vi "AlliGator Load IRFs & Fit Data (Map) HDF5 File v0.6.vi"(8 "Error In":errorcluster, 9 "File Type & Version only":bool, 11 "File Path":path) -> (0 "error out":errorcluster, 1 "Data Description":string, 2 "Decay Fit Options & Parameters":T1={"SYNC Period"=0.0, "Fit Options"={"Show Fit Residuals"=FALSE, "Fit Model"=enum."1-Exponential", "Residual Type"=enum."Standard", "Max Decay Percentile"=0.0, "Min Decay Percentile"=0.0, "Show Full Decay"=FALSE, "Weights"=enum."Unweighted", "Fitting Method"=enum."Least Square", "Compute Parameter Uncertainties"=FALSE, "Periodic Boundaries"=FALSE, "Model Calculation"=enum."Simulation", "Period"=0.0, "Termination Criteria"={"Max Iterations"=0, "Max Function Calls"=0, "Max Time"=0.0, "Function Tolerance"=0.0, "Parameter Tolerance"=0.0, "Gradient Tolerance"=0.0, "Min Lambda"=0.0, "Max Lambda"=0.0, "Initial Tick Count"=0}, "Offset Resolution"=0.0, "Use Local IRF"=FALSE, "Fitting Algorithm"=enum."Levenberg-Marquardt", "Show Confidence Interval "=TRUE, "Confidence Level"=95.0}, "Fit Parameter Constraints"=[], "MLE Baseline Offset"=0.0, "MLE Baseline Offset Type"=enum."Absolute"} {"Fit Options"."Confidence Level" min=0.0 max=100.0; "Fit Options"."Offset Resolution" min=0.0; "Fit Options"."Period" min=0.0; "Fit Options"."Min Decay Percentile" min=0.0 max=1.0; "Fit Options"."Max Decay Percentile" min=0.0 max=100.0; "Fit Parameter Constraints"."Max Value" format="%#.3g"; "Fit Parameter Constraints"."Min Value" format="%#.3g"}, 3 "IRFs & Fit Data Map v3":T13 {"Fit Options: Decay Preprocessing Parameters"."# Folds" min=1}, 4 "[Multiple Decays Fit Parameters SDV]":dbl[][](array[numeric]), 5 "File Version":string, 7 "File Type":string)   [LabVIEW 2021, in "AlliGator Decay Fit Parameter Map.lvlib"]
doc: "Loads Decay Fit Parameter Map and associated metadata."
uses:
  AlliGator Decay Fit Parameter Map.lvlib
  Fits/IRF(X)PSED/Decay Fit Parameters & Derived Quantities List v2.ctl
  Decay Analysis/Decay Preprocessing/AlliGator Decay Preprocessing Parameters.ctl
  Graphs/XY Graph/XY Graph Plot Shift Parameters.ctl
  Graphs/XY Graph/XY Graph Plot Shift Method.ctl
  AlliGator Decay Fit Options & Parameters v3.ctl
  Fits/IRF(X)PSED/Decay Fit Options v3.ctl
  Fits/Decay Convolution/Decay Model.ctl
  Fits/Residual Type.ctl
  Fits/IRF(X)PSED/Fit Weights Type.ctl
  Fits/Non-linear Fitting Method v2.ctl
  Fits/Fit Calculation Method.ctl
  Fits/Non-linear Fitting Algorithm.ctl
  Decay Analysis/Decay Fit/AlliGator Decay Fit Parameter Constraints 2.ctl
  Fits/IRF(X)PSED/Decay Fit Parameters In List.ctl
  Fits/IRF(X)PSED/MLE Baseline Offset Type.ctl
  Fits/IRF(X)PSED/Decay Fit Options v1.ctl
  Fits/Non-linear Fitting Method v1.ctl
  AlliGator IRFs & Fit Data v1.ctl
  Decay Analysis/Decay Fit/AlliGator Decay Fit Options & Parameters v1.ctl
  AlliGator Decay Fit Options & Parameters v2.ctl
  Fits/IRF(X)PSED/Decay Fit Options v2.ctl
  <vilib>/addons/h5labview2/base/lib_path.vi
  <vilib>/addons/h5labview2/base/H5Equery.vi
  <vilib>/addons/h5labview2/base/hid_t.ctl
  <vilib>/addons/h5labview2/dataset/H5Dread.llb/H5Dread.xnode
  <vilib>/addons/h5labview2/file/H5F.lvlib
  <vilib>/addons/h5labview2/group/H5G.lvlib
  Time/Time.lvlib
  Fits/Fits.lvlib
  Strings/Strings.lvlib
  Decay Analysis/Decay Fit/AlliGator Decay Fit.lvlib
  Graphs/XY Graph/XY Graph Add-Ons.lvlib
  Decay Analysis/Decay Preprocessing/AlliGator Decay Preprocessing.lvlib
  AlliGator IRFs & Fit Data v2.ctl
  AlliGator IRFs & Fit Data v3.ctl
panel:
  in  "Fit Parameter":T12(ring)
  out "elapsed (relative) seconds":dbl
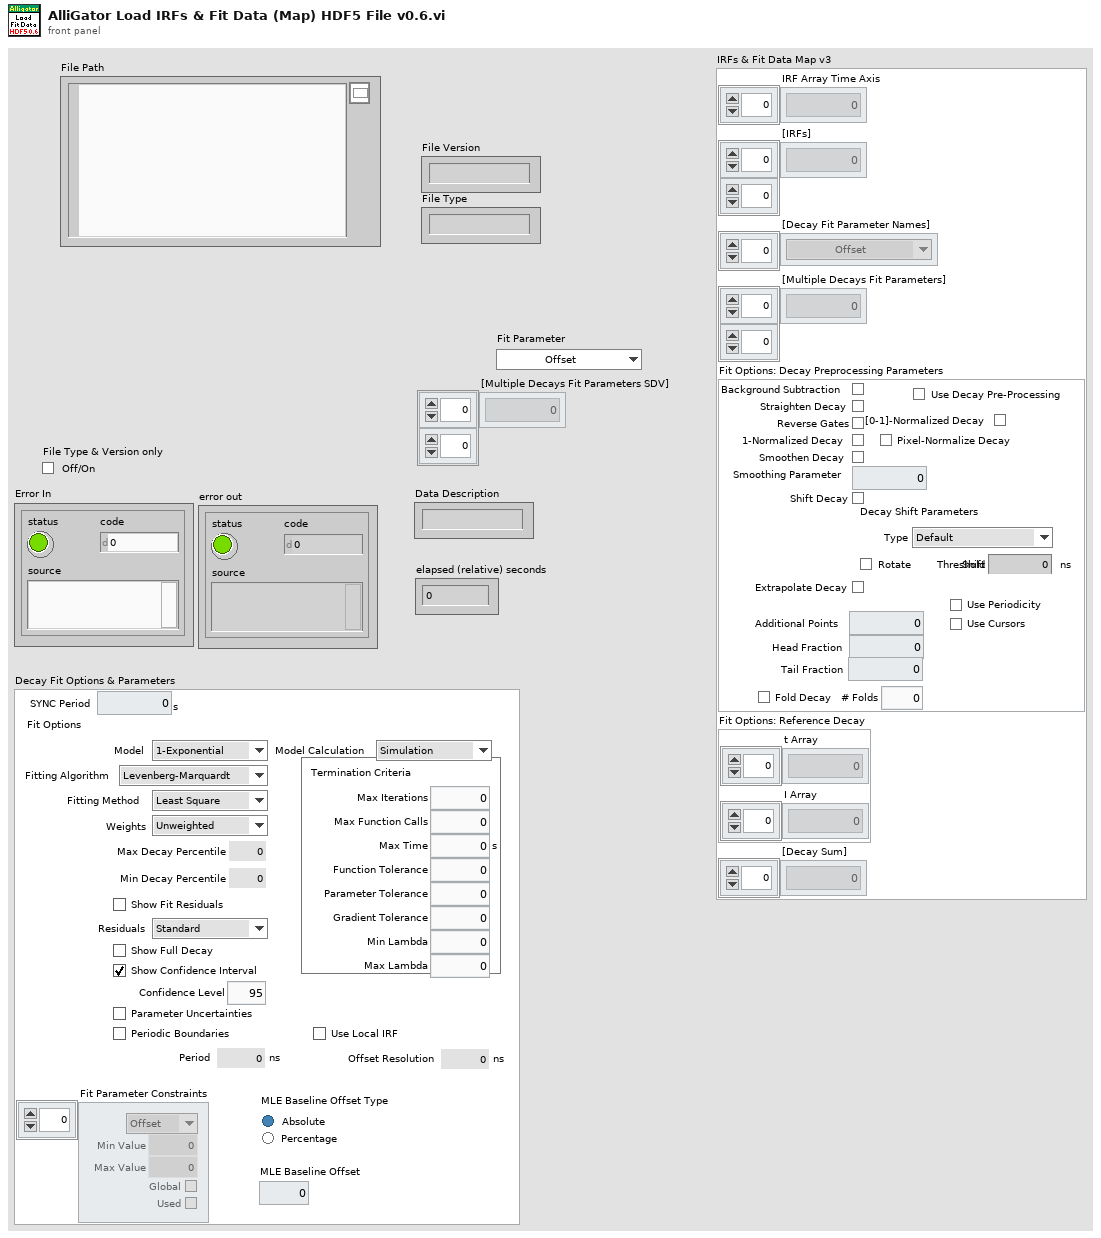
[diagram p1: front panel]
types:
  T1 = typedef "AlliGator Decay Fit Parameter Map.lvlib/AlliGator Decay Fit Options & Parameters v3.ctl" = cluster{"SYNC Period":dbl[unit], "Fit Options":T2, "Fit Parameter Constraints":T9[], "MLE Baseline Offset":dbl, "MLE Baseline Offset Type":T11}
  T2 = typedef "Fits.lvlib/Decay Fit Options v3.ctl" = cluster{"Show Fit Residuals":bool, "Fit Model":T3, "Residual Type":T4, "Max Decay Percentile":dbl, "Min Decay Percentile":dbl, "Show Full Decay":bool, "Weights":T5, "Fitting Method":T6, "Compute Parameter Uncertainties":bool, "Periodic Boundaries":bool, "Model Calculation":T7, "Period":dbl[unit], "Termination Criteria":cluster{"Max Iterations":i32, "Max Function Calls":i32, "Max Time":dbl[unit], "Function Tolerance":dbl, "Parameter Tolerance":dbl, "Gradient Tolerance":dbl, "Min Lambda":dbl, "Max Lambda":dbl, "Initial Tick Count":u32}, "Offset Resolution":dbl[unit], "Use Local IRF":bool, "Fitting Algorithm":T8, "Show Confidence Interval ":bool, "Confidence Level":dbl}
  T3 = typedef "Fits.lvlib/Decay Model.ctl" = enum16{"1-Exponential", "2-Exponentials"}
  T4 = typedef "Fits.lvlib/Residual Type.ctl" = enum16{"Standard", "Normalized", "Reduced"}
  T5 = typedef "Fits.lvlib/Fit Weights Type.ctl" = enum16{"Unweighted", "1/Variance", "Best of All"}
  T6 = typedef "Fits.lvlib/Non-linear Fitting Method v2.ctl" = enum16{"Least Square", "Least Absolute Residual", "Bisquare", "MLE", "-", "Best of All"}
  T7 = typedef "Fits.lvlib/Fit Calculation Method.ctl" = enum16{"Simulation", "Convolution", "Integration"}
  T8 = typedef "Fits.lvlib/Non-linear Fitting Algorithm.ctl" = enum16{"Levenberg-Marquardt", "Trust-Region Dogleg"}
  T9 = typedef "AlliGator Decay Fit.lvlib/AlliGator Decay Fit Parameter Constraints 2.ctl" = cluster{"Fit Parameter":T10, "Min Value":dbl, "Max Value":dbl, "Global":bool, "Used":bool}
  T10 = typedef "Fits.lvlib/Decay Fit Parameters In List.ctl" = enum16{"Offset", "Baseline", "A_1", "tau_1", "A_2", "tau_2"}
  T11 = typedef "Fits.lvlib/MLE Baseline Offset Type.ctl" = enum32{"Absolute", "Percentage"}
  T12 = enum16{"Offset", "Baseline", "A_1", "tau_1", "A_2", "tau_2", "<tau>_1", "f1_1", "f2_1", "<tau>_2", "f1_2", "f2_2", "-", "R^2", "Chi^2"}
  T13 = typedef "AlliGator Decay Fit Parameter Map.lvlib/AlliGator IRFs & Fit Data v3.ctl" = cluster{"IRF Array Time Axis":dbl[], "[IRFs]":dbl[][], "[Decay Fit Parameter Names]":T14[], "[Multiple Decays Fit Parameters]":dbl[][], "Fit Options: Decay Preprocessing Parameters":T15, "Fit Options: Reference Decay":cluster{"t Array":dbl[], "I Array":dbl[]}, "[Decay Sum]":dbl[]}
  T14 = typedef "Fits.lvlib/Decay Fit Parameters & Derived Quantities List v2.ctl" = enum16{"Offset", "Baseline", "A_1", "tau_1", "A_2", "tau_2", "<tau>_a", "f1_a", "f2_a", "<tau>_i", "f1_i", "f2_i", "-", "R^2", "Chi^2"}
  T15 = typedef "AlliGator Decay Preprocessing.lvlib/AlliGator Decay Preprocessing Parameters.ctl" = cluster{"Background Subtraction":bool, "Straighten Decay":bool, "Reverse Gates":bool, "1-Normalized Decay":bool, "Smoothen Decay":bool, "Smoothing Parameter":dbl, "Shift Decay":bool, "Decay Shift Parameters":T16, "Extrapolate Decay":bool, "Additional Points":u32, "Head Fraction":dbl, "Pixel-Normalize Decay":bool, "Use Periodicity":bool, "Use Cursors":bool, "Tail Fraction":dbl, "Use Decay Pre-Processing":bool, "Fold Decay":bool, "# Folds":u32, "[0-1]-Normalized Decay":bool}
  T16 = typedef "XY Graph Add-Ons.lvlib/XY Graph Plot Shift Parameters.ctl" = cluster{"Type":T17, "Shift":dbl[unit], "Threshold":dbl, "Rotate":bool}
  T17 = typedef "XY Graph Add-Ons.lvlib/XY Graph Plot Shift Method.ctl" = enum16{"Default", "CFD", "Threshold", "Cross-Correlation"}
  T18 = typedef "AlliGator Decay Fit.lvlib/AlliGator Decay Fit Options & Parameters v1.ctl" = cluster{"SYNC Period":dbl[unit], "Fit Options":T19, "Fit Parameter Constraints":T9[]}
  T19 = typedef "Fits.lvlib/Decay Fit Options v1.ctl" = cluster{"Show Fit Residuals":bool, "Fit Model":T3, "Residual Type":T4, "Max Decay Percentile":dbl, "Min Decay Percentile":dbl, "Show Full Decay":bool, "Weights":T5, "Fitting Method":T20, "Compute Parameter Uncertainties":bool, "Periodic Boundaries":bool, "Model Calculation":T7, "Period":dbl[unit], "Termination Criteria":cluster{"Max Iterations":i32, "Max Function Calls":i32, "Max Time":dbl[unit], "Function Tolerance":dbl, "Parameter Tolerance":dbl, "Gradient Tolerance":dbl, "Min Lambda":dbl, "Max Lambda":dbl, "Initial Tick Count":u32}, "Offset Resolution":dbl[unit], "Use Local IRF":bool, "Fitting Algorithm":T8}
  T20 = typedef "Fits.lvlib/Non-linear Fitting Method v1.ctl" = enum16{"Least Square", "Least Absolute Residual", "Bisquare", "-", "Best of All"}
  T21 = typedef "AlliGator Decay Fit Parameter Map.lvlib/AlliGator IRFs & Fit Data v1.ctl" = cluster{"IRF Array Time Axis":dbl[], "[IRF]":dbl[][], "[Decay Fit Parameter Name]":T14[], "[Multiple Decays Fit Parameters]":dbl[][]}
  T22 = typedef "AlliGator Decay Fit Parameter Map.lvlib/AlliGator IRFs & Fit Data v2.ctl" = cluster{"IRF Array Time Axis":dbl[], "[IRFs]":dbl[][], "[Decay Fit Parameter Names]":T14[], "[Multiple Decays Fit Parameters]":dbl[][], "Fit Options: Decay Preprocessing Parameters":T15, "Fit Options: Reference Decay":cluster{"t Array":dbl[], "I Array":dbl[]}}
  T23 = typedef "AlliGator Decay Fit Parameter Map.lvlib/AlliGator Decay Fit Options & Parameters v2.ctl" = cluster{"SYNC Period":dbl[unit], "Fit Options":T24, "Fit Parameter Constraints":T9[], "MLE Baseline Offset":dbl, "MLE Baseline Offset Type":T11}
  T24 = typedef "Fits.lvlib/Decay Fit Options v2.ctl" = cluster{"Show Fit Residuals":bool, "Fit Model":T3, "Residual Type":T4, "Max Decay Percentile":dbl, "Min Decay Percentile":dbl, "Show Full Decay":bool, "Weights":T5, "Fitting Method":T6, "Compute Parameter Uncertainties":bool, "Periodic Boundaries":bool, "Model Calculation":T7, "Period":dbl[unit], "Termination Criteria":cluster{"Max Iterations":i32, "Max Function Calls":i32, "Max Time":dbl[unit], "Function Tolerance":dbl, "Parameter Tolerance":dbl, "Gradient Tolerance":dbl, "Min Lambda":dbl, "Max Lambda":dbl, "Initial Tick Count":u32}, "Offset Resolution":dbl[unit], "Use Local IRF":bool, "Fitting Algorithm":T8}
  T25 = typedef "hid_t.ctl" = i64
  T26 = cluster{"Laser Period":dbl[unit], "Fit Options":T19, "Fit Parameter Constraints":T9[]}
  T27 = cluster{"IRF Array Time Axis":dbl[], "[IRF]":dbl[][], "[Decay Fit Parameter Name]":T14[], "[Multiple Decays Fit Parameters]":dbl[][]}
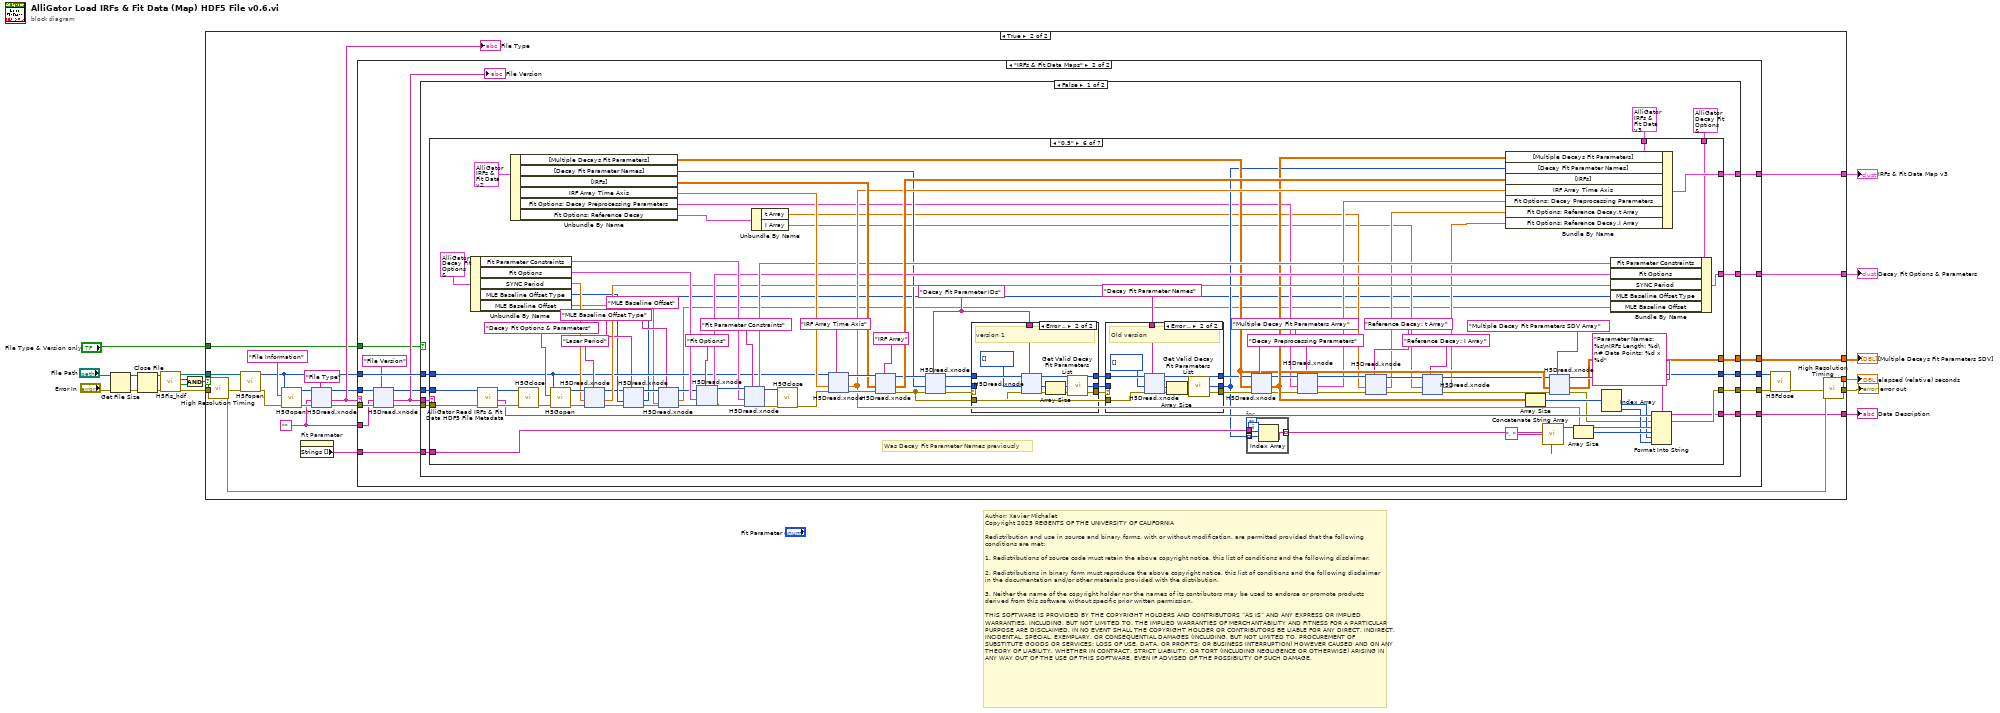
[diagram p0: block diagram]
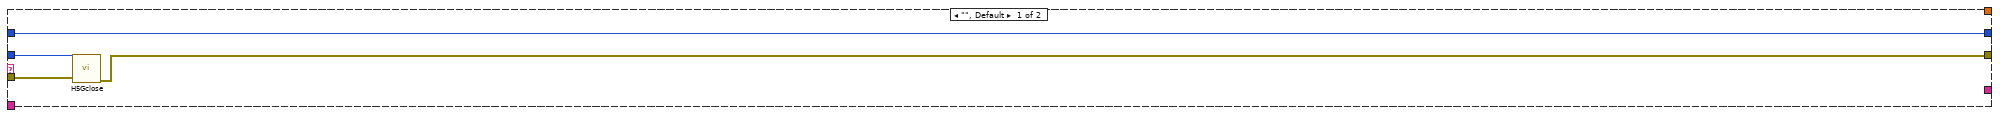
[diagram p3: hidden frame]
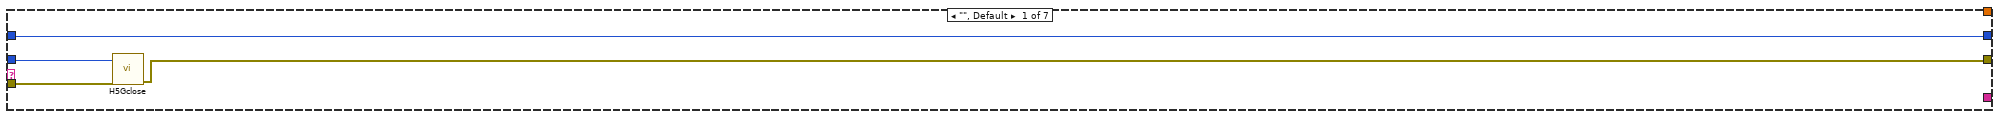
[diagram p4: hidden frame]
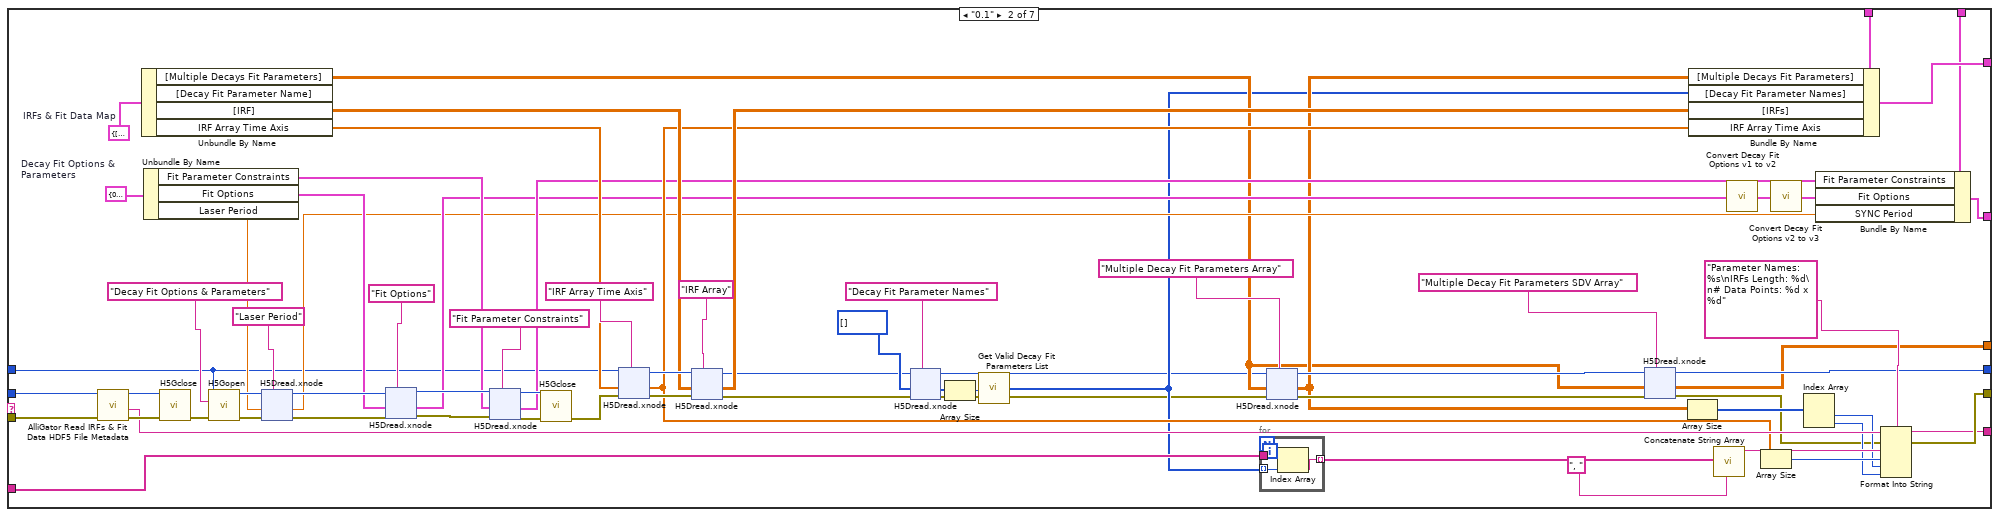
[diagram p5: hidden frame]
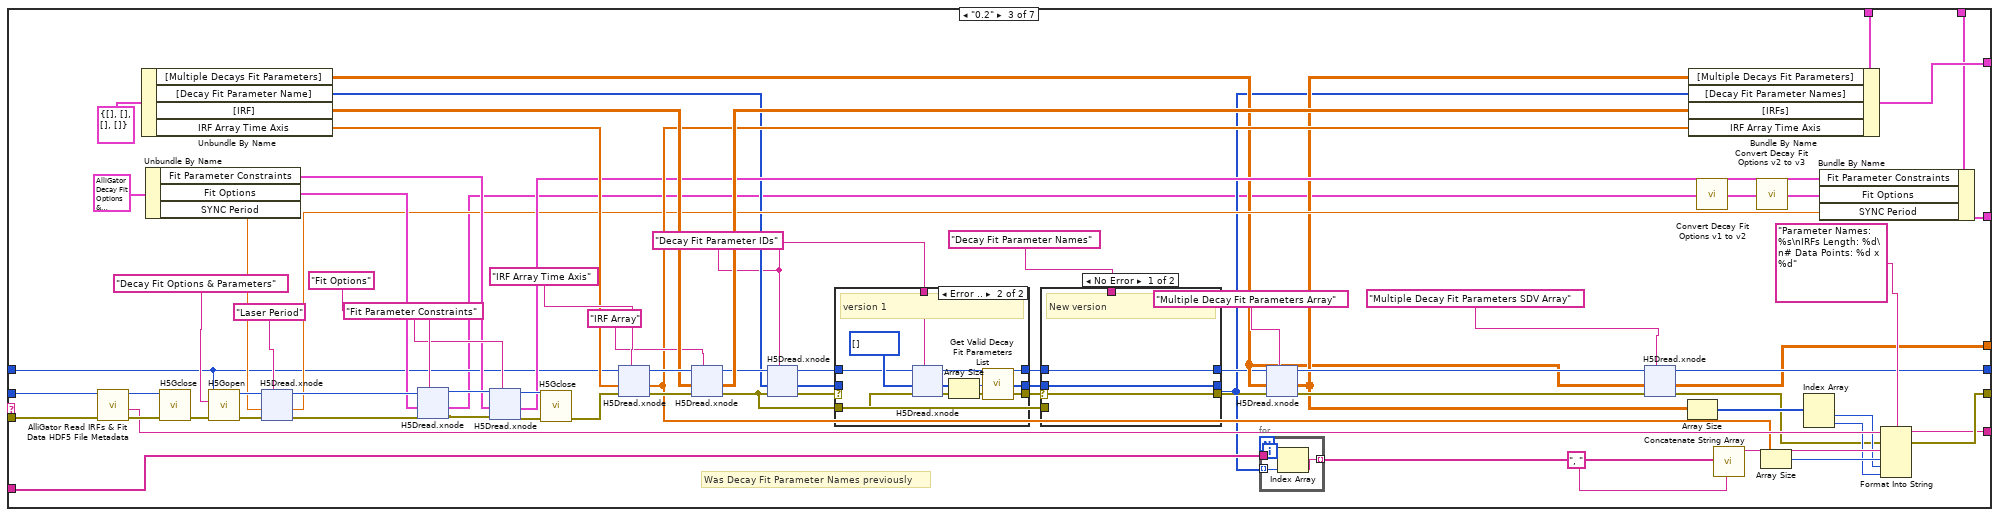
[diagram p6: hidden frame]
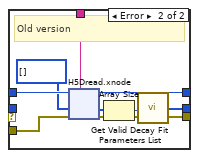
[diagram p8: hidden frame]
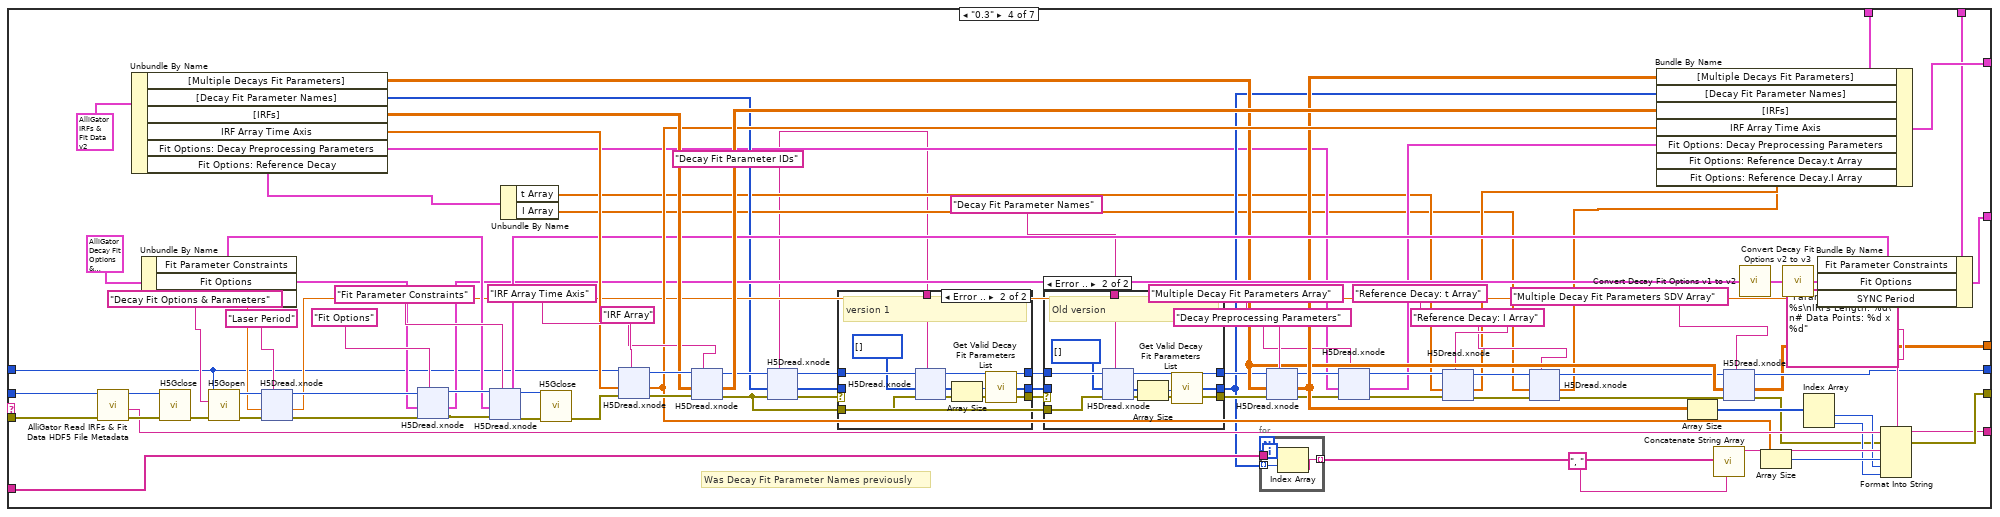
[diagram p9: hidden frame]
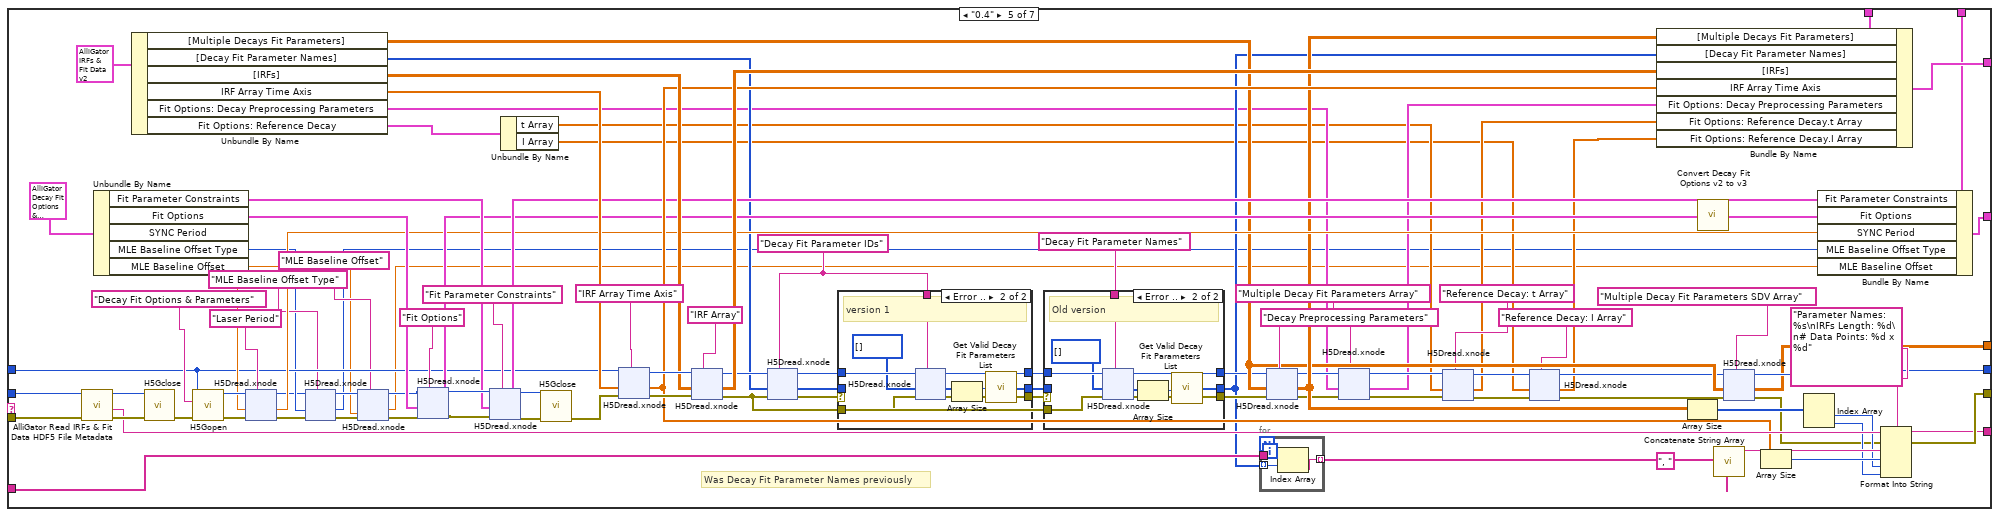
[diagram p12: hidden frame]
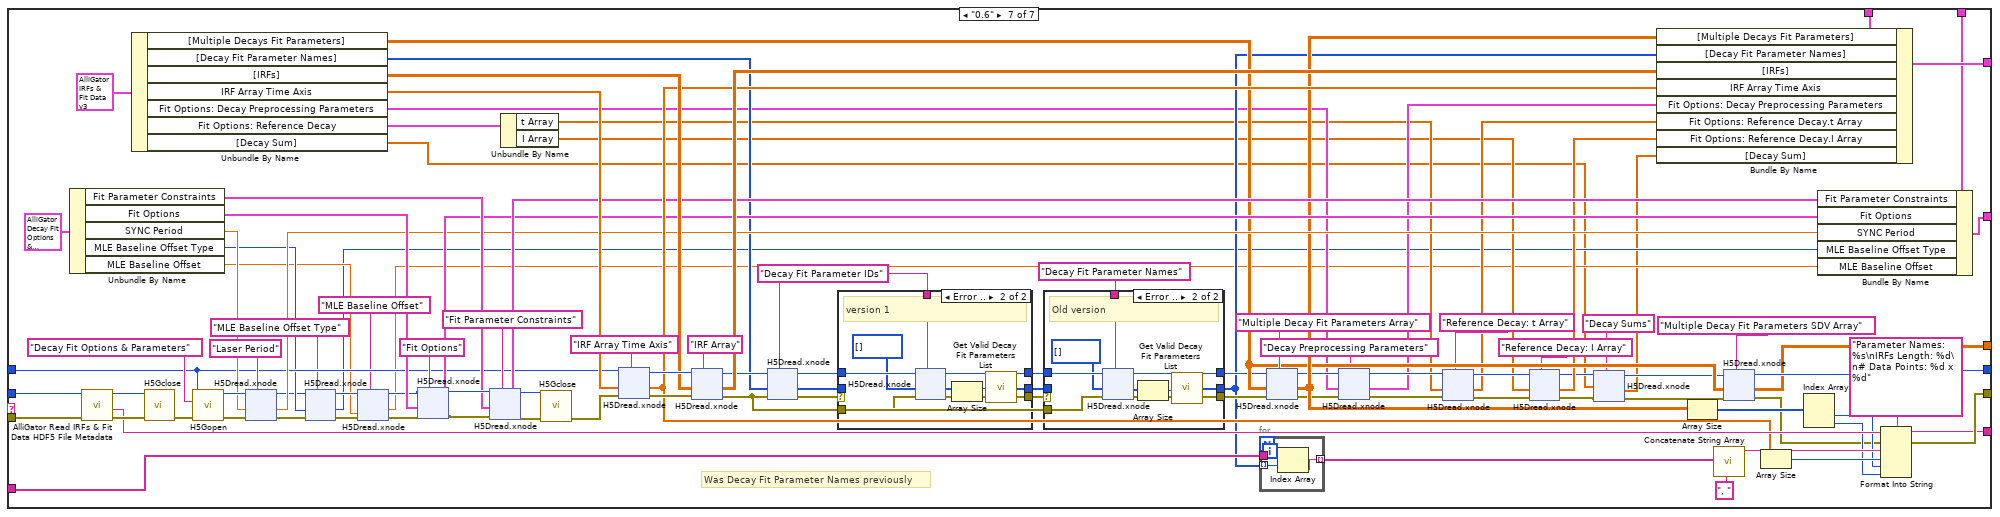
[diagram p17: hidden frame]
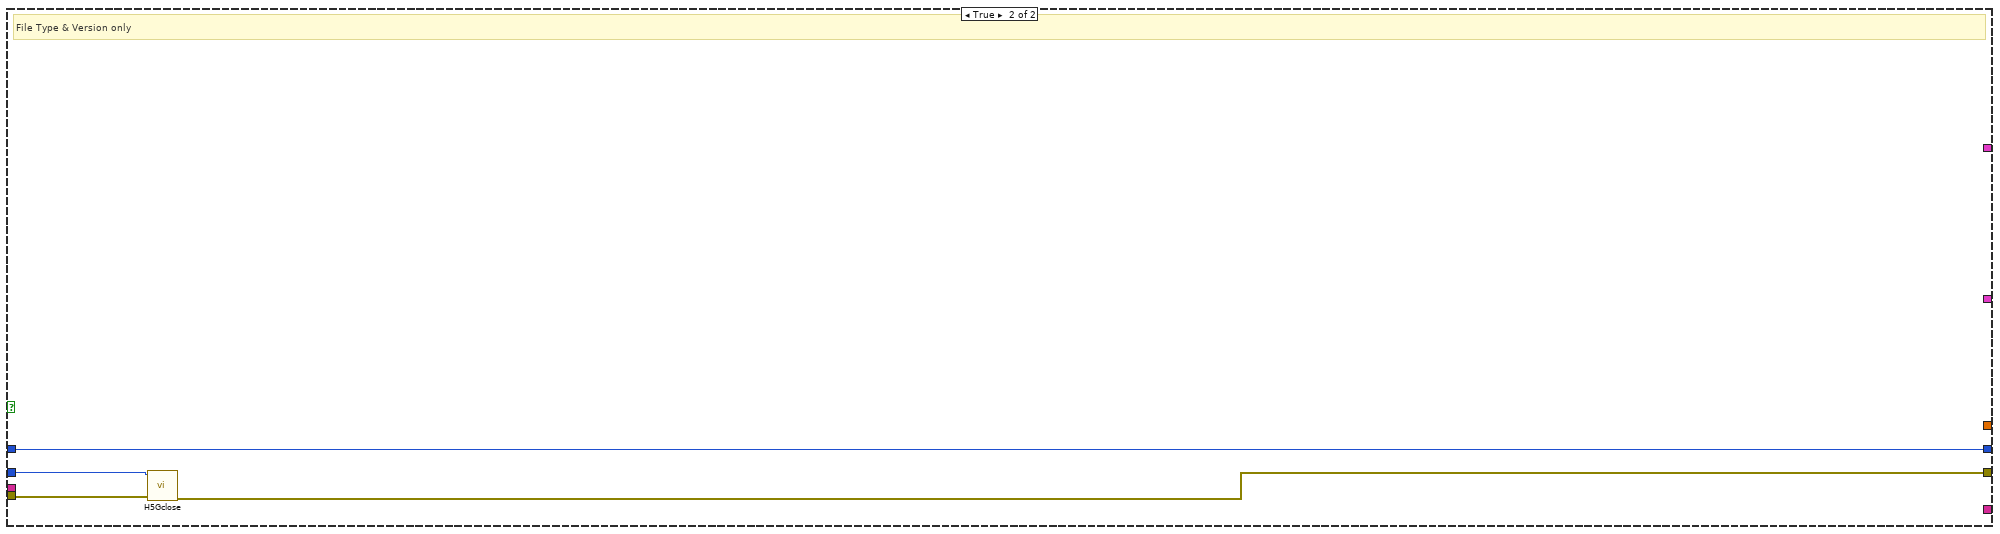
[diagram p20: hidden frame]
diagram:
  # "Author: Xavier Michalet\nCopyright 2025 REGENTS OF THE UNIVERSITY OF CALIFORNIA\n\nRedistribution and use in source and binary forms, with or without modification, are permitted provided that the following conditions are met:\n\n1. Redistributions of source code must retain the above copyright notice, this list of conditions and the following disclaimer.\n\n2. Redistributions in binary form must reproduce the above copyright notice, this list of conditions and the following disclaimer in the documentation and/or other materials provided with the distribution.\n\n3. Neither the name of the copyright holder nor the names of its contributors may be used to endorse or promote products derived from this software without specific prior written permission.\n\nTHIS SOFTWARE IS PROVIDED BY THE COPYRIGHT HOLDERS AND CONTRIBUTORS “AS IS” AND ANY EXPRESS OR IMPLIED WARRANTIES, INCLUDING, BUT NOT LIMITED TO, THE IMPLIED WARRANTIES OF MERCHANTABILITY AND FITNESS FOR A PARTICULAR PURPOSE ARE DISCLAIMED. IN NO EVENT SHALL THE COPYRIGHT HOLDER OR CONTRIBUTORS BE LIABLE FOR ANY DIRECT, INDIRECT, INCIDENTAL, SPECIAL, EXEMPLARY, OR CONSEQUENTIAL DAMAGES (INCLUDING, BUT NOT LIMITED TO, PROCUREMENT OF SUBSTITUTE GOODS OR SERVICES; LOSS OF USE, DATA, OR PROFITS; OR BUSINESS INTERRUPTION) HOWEVER CAUSED AND ON ANY THEORY OF LIABILITY, WHETHER IN CONTRACT, STRICT LIABILITY, OR TORT (INCLUDING NEGLIGENCE OR OTHERWISE) ARISING IN ANY WAY OUT OF THE USE OF THIS SOFTWARE, EVEN IF ADVISED OF THE POSSIBILITY OF SUCH DAMAGE."
  n1 = Get File Size(file="File Path", error in="Error In") -> (refnum out=w9:refnum<file>, 0:w10:errorcluster)  [unwired: 1 out]
  n2 = Close File(refnum=w9, error in=w10) -> (path=w8:path, error out=w7:errorcluster)
  n3 = call <vilib>:"H5Fis_hdf.vi"("error in (no error)"=w7, "path in"=w8) -> ("error out"=w14:errorcluster, "valid?"=w17:bool, "exists?"=w18:bool, "path out"=w15:path)  [unwired: 6 in]
  n4 = And(x=w18, y=w17) -> (x .and. y?=w16:bool)
  n5 = case shown="True" w16 {
    tunnel: w15 -> [_ w27]
    tunnel: w14 -> [w19 w44]
    tunnel: [w19 w39] -> w13
    tunnel: [_ w37] -> w6
    tunnel: [_ w26] -> w5
    tunnel: [_ w24] -> w4
    tunnel: [_ w22] -> w3
    tunnel: "File Type & Version only" -> [_ w21]
    tunnel: [_ w20] -> w1
    frame False {
    }
    frame True {
      w28 = ""
      n6 = call "High Resolution Timing.vi"("Error In"=w44) -> ("elapsed (relative) seconds"=w38:dbl, "Error Out"=w40:errorcluster)  [unwired: 16 in, 1 out]
      n7 = call <vilib>:"H5Fopen.vi"("error in (no error)"=w40, "path"=w27) -> ("error out"=w36:errorcluster, "ref out"=w31:T25)  [unwired: 8 in]
      n8 = call <vilib>:"H5Gopen.vi"("error in (no error)"=w36, "name"="File Information" ("dataset name (this)"), "ref in"=w31) -> ("error out"=w34:errorcluster, "group out"=w33:T25)  [unwired: 7 in]
      n9 = property on="Fit Parameter" class="Enum (strict)"() -> ("Strings []"=w23:string[])  [unwired: 2 in, 2 out]
      n10 = xnode "H5Dread.xnode"("dataset name (this)"="File Type", "error in (no error)"=w34, "default"=w28, "ref in"=w33) -> ("error out"=w30:errorcluster, "data"=w43:string, "ref out"=w29:T25)  [unwired: 2 in, 1 out]
      "File Type" <- w43
      n11 = case shown="\"IRFs & Fit Data Maps\"" w43 {
        tunnel: [w48 w64] -> w42
        tunnel: [w45 w57] -> w41
        tunnel: w31 -> [w48 w63]
        tunnel: w30 -> [w47 w61]
        tunnel: w28 -> [_ w60]
        tunnel: w29 -> [w46 w59]
        tunnel: [_ w56] -> w26
        tunnel: [_ w53] -> w24
        tunnel: w23 -> [_ w52]
        tunnel: [_ w51] -> w22
        tunnel: w21 -> [_ w50]
        tunnel: [_ w49] -> w20
        frame "", Default {
          n12 = call <vilib>:"H5Gclose.vi"("error in (no error)"=w47, "group in"=w46) -> ("error out"=w45:errorcluster)  [unwired: 9 in]
        }
        frame "IRFs & Fit Data Maps" {
          n13 = xnode "H5Dread.xnode"("dataset name (this)"="File Version", "error in (no error)"=w61, "default"=w60, "ref in"=w59) -> ("error out"=w55:errorcluster, "data"=w58:string, "ref out"=w54:T25)  [unwired: 2 in, 1 out]
          "File Version" <- w58
          n14 = case shown="False" w50 {
            tunnel: [w77 w1918] -> w64
            tunnel: w63 -> [w76 w1918]
            tunnel: w58 -> [w75 _]
            tunnel: [w74 w1917] -> w57
            tunnel: [w73 _] -> w56
            tunnel: w55 -> [w72 w1920]
            tunnel: w54 -> [w71 w1919]
            tunnel: [w70 _] -> w53
            tunnel: w52 -> [w69 _]
            tunnel: [w68 _] -> w51
            tunnel: [w67 _] -> w49
            frame False {
              n15 = case shown="\"0.5\"" w75 {
                tunnel: w76 -> [w81 w103 w302 w570 w894 w1245 w1601]
                tunnel: [w81 w99 w298 w568 w892 w1243 w1599] -> w77
                tunnel: [w78 w138 w336 w605 w927 w1278 w1634] -> w74
                tunnel: [_ w143 w341 w610 w932 w1283 w1639] -> w73
                tunnel: w72 -> [w80 w141 w339 w608 w930 w1281 w1637]
                tunnel: w71 -> [w79 w142 w340 w609 w931 w1282 w1638]
                tunnel: [_ w137 w335 w604 w926 w1277 w1633] -> w70
                tunnel: w69 -> [_ w134 w332 w601 w923 w1274 w1630]
                tunnel: [_ w104 w303 w571 w895 w1246 w1602] -> w68
                tunnel: [_ w95 w294 w564 w888 w1239 w1595] -> w67
                tunnel: T13 {"IRF Array Time Axis"=[], "[IRFs]"=[], "[Decay Fit Parameter Names]"=[], "[Multiple Decays Fit Parameters]"=[], "Fit Options: Decay Preprocessing Parameters"={"Background Subtraction"=FALSE, "Straighten Decay"=FALSE, "Reverse Gates"=FALSE, "1-Normalized Decay"=FALSE, "Smoothen Decay"=FALSE, "Smoothing Parameter"=0.0, "Shift Decay"=FALSE, "Decay Shift Parameters"={"Type"=enum."Default", "Shift"=0.0, "Threshold"=0.0, "Rotate"=FALSE}, "Extrapolate Decay"=FALSE, "Additional Points"=0, "Head Fraction"=0.0, "Pixel-Normalize Decay"=FALSE, "Use Periodicity"=FALSE, "Use Cursors"=FALSE, "Tail Fraction"=0.0, "Use Decay Pre-Processing"=FALSE, "Fold Decay"=FALSE, "# Folds"=0, "[0-1]-Normalized Decay"=FALSE}, "Fit Options: Reference Decay"={"t Array"=[], "I Array"=[]}, "[Decay Sum]"=[]} ("IRFs & Fit Data Map") -> [_ w94 w292 w558 w882 w1233 w1589]
                tunnel: T1 {"SYNC Period"=0.0, "Fit Options"={"Show Fit Residuals"=FALSE, "Fit Model"=enum."1-Exponential", "Residual Type"=enum."Standard", "Max Decay Percentile"=0.0, "Min Decay Percentile"=0.0, "Show Full Decay"=FALSE, "Weights"=enum."Unweighted", "Fitting Method"=enum."Least Square", "Compute Parameter Uncertainties"=FALSE, "Periodic Boundaries"=FALSE, "Model Calculation"=enum."Simulation", "Period"=0.0, "Termination Criteria"={"Max Iterations"=0, "Max Function Calls"=0, "Max Time"=0.0, "Function Tolerance"=0.0, "Parameter Tolerance"=0.0, "Gradient Tolerance"=0.0, "Min Lambda"=0.0, "Max Lambda"=0.0, "Initial Tick Count"=0}, "Offset Resolution"=0.0, "Use Local IRF"=FALSE, "Fitting Algorithm"=enum."Levenberg-Marquardt", "Show Confidence Interval "=TRUE, "Confidence Level"=95.0}, "Fit Parameter Constraints"=[], "MLE Baseline Offset"=0.0, "MLE Baseline Offset Type"=enum."Absolute"} ("Decay Fit Options & Parameters") -> [_ w84 w279 w531 w855 w1206 w1564]
                frame "", Default {
                  n16 = call <vilib>:"H5Gclose.vi"("error in (no error)"=w80, "group in"=w79) -> ("error out"=w78:errorcluster)  [unwired: 9 in]
                }
                frame "0.1" {
                  w108 = T26 {"Laser Period"=0.0, "Fit Options"={"Show Fit Residuals"=FALSE, "Fit Model"=enum."1-Exponential", "Residual Type"=enum."Standard", "Max Decay Percentile"=0.0, "Min Decay Percentile"=0.0, "Show Full Decay"=FALSE, "Weights"=enum."Unweighted", "Fitting Method"=enum."Least Square", "Compute Parameter Uncertainties"=FALSE, "Periodic Boundaries"=FALSE, "Model Calculation"=enum."Simulation", "Period"=0.0, "Termination Criteria"={"Max Iterations"=0, "Max Function Calls"=0, "Max Time"=0.0, "Function Tolerance"=0.0, "Parameter Tolerance"=0.0, "Gradient Tolerance"=0.0, "Min Lambda"=0.0, "Max Lambda"=0.0, "Initial Tick Count"=0}, "Offset Resolution"=0.0, "Use Local IRF"=FALSE, "Fitting Algorithm"=enum."Levenberg-Marquardt"}, "Fit Parameter Constraints"=[]}  # Decay Fit Options & Parameters
                  w148 = T27 {"IRF Array Time Axis"=[], "[IRF]"=[], "[Decay Fit Parameter Name]"=[], "[Multiple Decays Fit Parameters]"=[]}  # IRFs & Fit Data Map
                  n17 = call "AlliGator Read IRFs & Fit Data HDF5 File Metadata.vi"("error in (no error)"=w141, "ref in"=w142) -> ("error out"=w139:errorcluster, "File Metadata"=w136:string, "ref out"=w140:T25)  [unwired: 7 in]
                  n18 = Unbundle By Name(w148) -> ("[Multiple Decays Fit Parameters]"=w96:dbl[][], "[IRF]"=w147:dbl[][], "IRF Array Time Axis"=w149:dbl[])  [unwired: 1 out]
                  n19 = Unbundle By Name(w108) -> ("Fit Parameter Constraints"=w109:T9[], "Fit Options"=w110:T19, "Laser Period"=w111:dbl[unit])
                  n20 = call <vilib>:"H5Gclose.vi"("error in (no error)"=w139, "group in"=w140) -> ("error out"=w114:errorcluster)  [unwired: 9 in]
                  n21 = call <vilib>:"H5Gopen.vi"("error in (no error)"=w114, "name"="Decay Fit Options & Parameters" ("dataset name"), "ref in"=w103) -> ("error out"=w125:errorcluster, "group out"=w124:T25)  [unwired: 7 in]
                  n22 = xnode "H5Dread.xnode"("dataset name (this)"="Laser Period" ("dataset name"), "error in (no error)"=w125, "default"=w111, "ref in"=w124) -> ("error out"=w123:errorcluster, "data"=w105:dbl[unit], "ref out"=w120:T25)  [unwired: 2 in, 1 out]
                  n23 = xnode "H5Dread.xnode"("dataset name (this)"="Fit Options" ("dataset name"), "error in (no error)"=w123, "default"=w110, "ref in"=w120) -> ("error out"=w122:errorcluster, "data"=w106:T19, "ref out"=w119:i64)  [unwired: 2 in, 1 out]
                  n24 = xnode "H5Dread.xnode"("dataset name (this)"="Fit Parameter Constraints" ("dataset name"), "error in (no error)"=w122, "default"=w109, "ref in"=w119) -> ("error out"=w121:errorcluster, "data"=w107:T9[], "ref out"=w118:i64)  [unwired: 2 in, 1 out]
                  n25 = call <vilib>:"H5Gclose.vi"("error in (no error)"=w121, "group in"=w118) -> ("error out"=w113:errorcluster)  [unwired: 9 in]
                  n26 = xnode "H5Dread.xnode"("dataset name (this)"="IRF Array Time Axis" ("dataset name"), "error in (no error)"=w113, "default"=w149, "ref in"=w103) -> ("error out"=w152:errorcluster, "data"=w129:dbl[], "ref out"=w151:T25)  [unwired: 2 in, 1 out]
                  n27 = xnode "H5Dread.xnode"("dataset name (this)"="IRF Array" ("dataset name"), "error in (no error)"=w152, "default"=w147, "ref in"=w151) -> ("error out"=w92:errorcluster, "data"=w145:dbl[][], "ref out"=w87:T25)  [unwired: 2 in, 1 out]
                  n28 = xnode "H5Dread.xnode"("dataset name (this)"="Decay Fit Parameter Names" ("name"), "error in (no error)"=w92, "default"=u16[] [], "ref in"=w87) -> ("error out"=w85:errorcluster, "data"=w90:u16[], "ref out"=w86:i64)  [unwired: 2 in, 1 out]
                  n29 = Array Size(array=w90) -> (size(s)=w89:i32)
                  n30 = call "Get Valid Decay Fit Parameters List.vi"("Parameter ID Array Size"=w89) -> ("Parameter Name Array"=w88:T14[])
                  n31 = for {
                    tunnel: w134 -> [w230]
                    tunnel: [w229] -> w133 mode=indexing
                    tunnel: w88 -> [w228] mode=indexing
                    n32 = Index Array(array=w230, index=w228) -> (element=w229:string)
                  }
                  n33 = xnode "H5Dread.xnode"("dataset name (this)"="Multiple Decay Fit Parameters Array" ("name"), "error in (no error)"=w85, "default"=w96, "ref in"=w86) -> ("error out"=w102:errorcluster, "data"=w97:dbl[][], "ref out"=w100:T25)  [unwired: 2 in, 1 out]
                  n34 = xnode "H5Dread.xnode"("dataset name (this)"="Multiple Decay Fit Parameters SDV Array" ("name"), "error in (no error)"=w102, "default"=w96, "ref in"=w100) -> ("error out"=w101:errorcluster, "data"=w95:dbl[][], "ref out"=w99:T25)  [unwired: 2 in, 1 out]
                  n35 = Array Size(array=w97) -> (size(s)=w128:i32[])
                  n36 = Bundle By Name(cluster=w94, "[Multiple Decays Fit Parameters]"=w97, "[Decay Fit Parameter Names]"=w88, "[IRFs]"=w145, "IRF Array Time Axis"=w129) -> (w143:T13)
                  n37 = call "Concatenate String Array.vi"("Separator (TAB)"=", ", "String Array"=w133) -> ("Formatted String"=w131:string)  [unwired: 9 in]
                  n38 = call "Convert Decay Fit Options v1 to v2.vi"("Decay Fit Options v1"=w106) -> ("Decay Fit Options v2"=w83:T24)
                  n39 = Array Size(array=w129) -> (size(s)=w130:i32)
                  n40 = call "Convert Decay Fit Options v2 to v3.vi"("Decay Fit Options v2"=w83) -> ("Decay Fit Options v3"=w82:T2)
                  n41 = Index Array(array=w128) -> (element #1=w127:i32, element #2=w126:i32)  [unwired: 2 in]
                  n42 = Bundle By Name(cluster=w84, "Fit Parameter Constraints"=w107, "Fit Options"=w82, "SYNC Period"=w105) -> (w104:T1)
                  n43 = Format Into String(format string="Parameter Names: %s\nIRFs Length: %d\n# Data Points: %d x %d", initial string=w136, error in=w101, w131, w130, w127, w126) -> (resulting string=w137:string, error out=w138:errorcluster)
                }
                frame "0.2" {
                  w287 = "Decay Fit Parameter IDs" ("name")
                  # "Was Decay Fit Parameter Names previously"
                  n44 = call "AlliGator Read IRFs & Fit Data HDF5 File Metadata.vi"("error in (no error)"=w339, "ref in"=w340) -> ("error out"=w337:errorcluster, "File Metadata"=w334:string, "ref out"=w338:T25)  [unwired: 7 in]
                  n45 = Unbundle By Name(T21 {"IRF Array Time Axis"=[], "[IRF]"=[], "[Decay Fit Parameter Name]"=[], "[Multiple Decays Fit Parameters]"=[]} ("IRFs & Fit Data Map")) -> ("[Multiple Decays Fit Parameters]"=w295:dbl[][], "[Decay Fit Parameter Name]"=w293:T14[], "[IRF]"=w346:dbl[][], "IRF Array Time Axis"=w348:dbl[])
                  n46 = Unbundle By Name(T18 {"SYNC Period"=0.0, "Fit Options"={"Show Fit Residuals"=FALSE, "Fit Model"=enum."1-Exponential", "Residual Type"=enum."Standard", "Max Decay Percentile"=0.0, "Min Decay Percentile"=0.0, "Show Full Decay"=FALSE, "Weights"=enum."Unweighted", "Fitting Method"=enum."Least Square", "Compute Parameter Uncertainties"=FALSE, "Periodic Boundaries"=FALSE, "Model Calculation"=enum."Simulation", "Period"=0.0, "Termination Criteria"={"Max Iterations"=0, "Max Function Calls"=0, "Max Time"=0.0, "Function Tolerance"=0.0, "Parameter Tolerance"=0.0, "Gradient Tolerance"=0.0, "Min Lambda"=0.0, "Max Lambda"=0.0, "Initial Tick Count"=0}, "Offset Resolution"=0.0, "Use Local IRF"=FALSE, "Fitting Algorithm"=enum."Levenberg-Marquardt"}, "Fit Parameter Constraints"=[]} ("Decay Fit Options & Parameters")) -> ("Fit Parameter Constraints"=w307:T9[], "Fit Options"=w308:T19, "SYNC Period"=w309:dbl[unit])
                  n47 = call <vilib>:"H5Gclose.vi"("error in (no error)"=w337, "group in"=w338) -> ("error out"=w312:errorcluster)  [unwired: 9 in]
                  n48 = call <vilib>:"H5Gopen.vi"("error in (no error)"=w312, "name"="Decay Fit Options & Parameters" ("dataset name"), "ref in"=w302) -> ("error out"=w323:errorcluster, "group out"=w322:T25)  [unwired: 7 in]
                  n49 = xnode "H5Dread.xnode"("dataset name (this)"="Laser Period" ("dataset name"), "error in (no error)"=w323, "default"=w309, "ref in"=w322) -> ("error out"=w321:errorcluster, "data"=w304:dbl[unit], "ref out"=w318:T25)  [unwired: 2 in, 1 out]
                  n50 = xnode "H5Dread.xnode"("dataset name (this)"="Fit Options" ("dataset name"), "error in (no error)"=w321, "default"=w308, "ref in"=w318) -> ("error out"=w320:errorcluster, "data"=w278:T19, "ref out"=w317:i64)  [unwired: 2 in, 1 out]
                  n51 = xnode "H5Dread.xnode"("dataset name (this)"="Fit Parameter Constraints" ("dataset name"), "error in (no error)"=w320, "default"=w307, "ref in"=w317) -> ("error out"=w319:errorcluster, "data"=w305:T9[], "ref out"=w316:T25)  [unwired: 2 in, 1 out]
                  n52 = call <vilib>:"H5Gclose.vi"("error in (no error)"=w319, "group in"=w316) -> ("error out"=w311:errorcluster)  [unwired: 9 in]
                  n53 = xnode "H5Dread.xnode"("dataset name (this)"="IRF Array Time Axis" ("dataset name"), "error in (no error)"=w311, "default"=w348, "ref in"=w302) -> ("error out"=w351:errorcluster, "data"=w327:dbl[], "ref out"=w350:T25)  [unwired: 2 in, 1 out]
                  n54 = xnode "H5Dread.xnode"("dataset name (this)"="IRF Array" ("dataset name"), "error in (no error)"=w351, "default"=w346, "ref in"=w350) -> ("error out"=w282:errorcluster, "data"=w344:dbl[][], "ref out"=w343:T25)  [unwired: 2 in, 1 out]
                  n55 = xnode "H5Dread.xnode"("dataset name (this)"=w287, "error in (no error)"=w282, "default"=w293, "ref in"=w343) -> ("error out"=w283:errorcluster, "data"=w281:T14[], "ref out"=w288:i64)  [unwired: 2 in, 1 out]
                  n56 = case shown="Error .." w283 {
                    selector: w283 -> [w354 _]
                    tunnel: [w353 w363] -> w291
                    tunnel: [w354 w362] -> w290
                    tunnel: [w352 w360] -> w289
                    tunnel: w288 -> [w353 w357]
                    tunnel: w287 -> [_ w356]
                    tunnel: w282 -> [_ w355]
                    tunnel: w281 -> [w352 _]
                    frame No Error {
                      # "New version"
                    }
                    frame Error {
                      # "version 1"
                      n57 = xnode "H5Dread.xnode"("dataset name (this)"=w356, "error in (no error)"=w355, "default"=u16[] [], "ref in"=w357) -> ("error out"=w362:errorcluster, "data"=w359:u16[], "ref out"=w363:i64)  [unwired: 2 in, 1 out]
                      n58 = Array Size(array=w359) -> (size(s)=w358:i32)
                      n59 = call "Get Valid Decay Fit Parameters List.vi"("Parameter ID Array Size"=w358) -> ("Parameter Name Array"=w360:T14[])
                    }
                  }
                  n60 = case shown="No Error" w290 {
                    selector: w290 -> [w380 _]
                    tunnel: w291 -> [w381 w390]
                    tunnel: [w381 w389] -> w284
                    tunnel: [w380 w388] -> w285
                    tunnel: w289 -> [w379 _]
                    tunnel: [w379 w387] -> w280
                    tunnel: "Decay Fit Parameter Names" ("name") -> [_ w383]
                    tunnel: w282 -> [_ w382]
                    frame No Error {
                      # "New version"
                    }
                    frame Error {
                      # "Old version"
                      n61 = xnode "H5Dread.xnode"("dataset name (this)"=w383, "error in (no error)"=w382, "default"=u16[] [], "ref in"=w390) -> ("error out"=w388:errorcluster, "data"=w385:u16[], "ref out"=w389:i64)  [unwired: 2 in, 1 out]
                      n62 = Array Size(array=w385) -> (size(s)=w384:i32)
                      n63 = call "Get Valid Decay Fit Parameters List.vi"("Parameter ID Array Size"=w384) -> ("Parameter Name Array"=w387:T14[])
                    }
                  }
                  n64 = for {
                    tunnel: w332 -> [w483]
                    tunnel: [w482] -> w331 mode=indexing
                    tunnel: w280 -> [w481] mode=indexing
                    n65 = Index Array(array=w483, index=w481) -> (element=w482:string)
                  }
                  n66 = xnode "H5Dread.xnode"("dataset name (this)"="Multiple Decay Fit Parameters Array" ("name"), "error in (no error)"=w285, "default"=w295, "ref in"=w284) -> ("error out"=w301:errorcluster, "data"=w296:dbl[][], "ref out"=w299:T25)  [unwired: 2 in, 1 out]
                  n67 = xnode "H5Dread.xnode"("dataset name (this)"="Multiple Decay Fit Parameters SDV Array" ("name"), "error in (no error)"=w301, "default"=w295, "ref in"=w299) -> ("error out"=w300:errorcluster, "data"=w294:dbl[][], "ref out"=w298:T25)  [unwired: 2 in, 1 out]
                  n68 = Array Size(array=w296) -> (size(s)=w326:i32[])
                  n69 = Bundle By Name(cluster=w292, "[Multiple Decays Fit Parameters]"=w296, "[Decay Fit Parameter Names]"=w280, "[IRFs]"=w344, "IRF Array Time Axis"=w327) -> (w341:T13)
                  n70 = call "Convert Decay Fit Options v1 to v2.vi"("Decay Fit Options v1"=w278) -> ("Decay Fit Options v2"=w277:T24)
                  n71 = call "Concatenate String Array.vi"("Separator (TAB)"=", ", "String Array"=w331) -> ("Formatted String"=w329:string)  [unwired: 9 in]
                  n72 = call "Convert Decay Fit Options v2 to v3.vi"("Decay Fit Options v2"=w277) -> ("Decay Fit Options v3"=w276:T2)
                  n73 = Array Size(array=w327) -> (size(s)=w328:i32)
                  n74 = Index Array(array=w326) -> (element #1=w325:i32, element #2=w324:i32)  [unwired: 2 in]
                  n75 = Bundle By Name(cluster=w279, "Fit Parameter Constraints"=w305, "Fit Options"=w276, "SYNC Period"=w304) -> (w303:T1)
                  n76 = Format Into String(format string="Parameter Names: %s\nIRFs Length: %d\n# Data Points: %d x %d", initial string=w334, error in=w300, w329, w328, w325, w324) -> (resulting string=w335:string, error out=w336:errorcluster)
                }
                frame "0.3" {
                  w538 = "Decay Fit Parameter IDs" ("name")
                  # "Was Decay Fit Parameter Names previously"
                  n77 = call "AlliGator Read IRFs & Fit Data HDF5 File Metadata.vi"("error in (no error)"=w608, "ref in"=w609) -> ("error out"=w606:errorcluster, "File Metadata"=w603:string, "ref out"=w607:T25)  [unwired: 7 in]
                  n78 = Unbundle By Name(T22 {"IRF Array Time Axis"=[], "[IRFs]"=[], "[Decay Fit Parameter Names]"=[], "[Multiple Decays Fit Parameters]"=[], "Fit Options: Decay Preprocessing Parameters"={"Background Subtraction"=FALSE, "Straighten Decay"=FALSE, "Reverse Gates"=FALSE, "1-Normalized Decay"=FALSE, "Smoothen Decay"=FALSE, "Smoothing Parameter"=0.0, "Shift Decay"=FALSE, "Decay Shift Parameters"={"Type"=enum."Default", "Shift"=0.0, "Threshold"=0.0, "Rotate"=FALSE}, "Extrapolate Decay"=FALSE, "Additional Points"=0, "Head Fraction"=0.0, "Pixel-Normalize Decay"=FALSE, "Use Periodicity"=FALSE, "Use Cursors"=FALSE, "Tail Fraction"=0.0, "Use Decay Pre-Processing"=FALSE, "Fold Decay"=FALSE, "# Folds"=0, "[0-1]-Normalized Decay"=FALSE}, "Fit Options: Reference Decay"={"t Array"=[], "I Array"=[]}} ("IRFs & Fit Data Map")) -> ("[Multiple Decays Fit Parameters]"=w565:dbl[][], "[Decay Fit Parameter Names]"=w559:T14[], "[IRFs]"=w615:dbl[][], "IRF Array Time Axis"=w617:dbl[], "Fit Options: Decay Preprocessing Parameters"=w546:T15, "Fit Options: Reference Decay"=w544:cluster{"t Array":dbl[], "I Array":dbl[]})
                  n79 = Unbundle By Name(T18 {"SYNC Period"=0.0, "Fit Options"={"Show Fit Residuals"=FALSE, "Fit Model"=enum."1-Exponential", "Residual Type"=enum."Standard", "Max Decay Percentile"=0.0, "Min Decay Percentile"=0.0, "Show Full Decay"=FALSE, "Weights"=enum."Unweighted", "Fitting Method"=enum."Least Square", "Compute Parameter Uncertainties"=FALSE, "Periodic Boundaries"=FALSE, "Model Calculation"=enum."Simulation", "Period"=0.0, "Termination Criteria"={"Max Iterations"=0, "Max Function Calls"=0, "Max Time"=0.0, "Function Tolerance"=0.0, "Parameter Tolerance"=0.0, "Gradient Tolerance"=0.0, "Min Lambda"=0.0, "Max Lambda"=0.0, "Initial Tick Count"=0}, "Offset Resolution"=0.0, "Use Local IRF"=FALSE, "Fitting Algorithm"=enum."Levenberg-Marquardt"}, "Fit Parameter Constraints"=[]} ("Decay Fit Options & Parameters")) -> ("Fit Parameter Constraints"=w576:T9[], "Fit Options"=w577:T19, "SYNC Period"=w578:dbl[unit])
                  n80 = call <vilib>:"H5Gclose.vi"("error in (no error)"=w606, "group in"=w607) -> ("error out"=w581:errorcluster)  [unwired: 9 in]
                  n81 = call <vilib>:"H5Gopen.vi"("error in (no error)"=w581, "name"="Decay Fit Options & Parameters" ("dataset name"), "ref in"=w570) -> ("error out"=w592:errorcluster, "group out"=w591:T25)  [unwired: 7 in]
                  n82 = xnode "H5Dread.xnode"("dataset name (this)"="Laser Period" ("dataset name"), "error in (no error)"=w592, "default"=w578, "ref in"=w591) -> ("error out"=w590:errorcluster, "data"=w572:dbl[unit], "ref out"=w587:T25)  [unwired: 2 in, 1 out]
                  n83 = xnode "H5Dread.xnode"("dataset name (this)"="Fit Options" ("dataset name"), "error in (no error)"=w590, "default"=w577, "ref in"=w587) -> ("error out"=w589:errorcluster, "data"=w573:T19, "ref out"=w586:i64)  [unwired: 2 in, 1 out]
                  n84 = xnode "H5Dread.xnode"("dataset name (this)"="Fit Parameter Constraints" ("dataset name"), "error in (no error)"=w589, "default"=w576, "ref in"=w586) -> ("error out"=w588:errorcluster, "data"=w574:T9[], "ref out"=w585:T25)  [unwired: 2 in, 1 out]
                  n85 = Unbundle By Name(w544) -> ("t Array"=w543:dbl[], "I Array"=w541:dbl[])
                  n86 = call <vilib>:"H5Gclose.vi"("error in (no error)"=w588, "group in"=w585) -> ("error out"=w580:errorcluster)  [unwired: 9 in]
                  n87 = xnode "H5Dread.xnode"("dataset name (this)"="IRF Array Time Axis" ("dataset name"), "error in (no error)"=w580, "default"=w617, "ref in"=w570) -> ("error out"=w620:errorcluster, "data"=w596:dbl[], "ref out"=w619:T25)  [unwired: 2 in, 1 out]
                  n88 = xnode "H5Dread.xnode"("dataset name (this)"="IRF Array" ("dataset name"), "error in (no error)"=w620, "default"=w615, "ref in"=w619) -> ("error out"=w533:errorcluster, "data"=w613:dbl[][], "ref out"=w612:T25)  [unwired: 2 in, 1 out]
                  n89 = xnode "H5Dread.xnode"("dataset name (this)"=w538, "error in (no error)"=w533, "default"=w559, "ref in"=w612) -> ("error out"=w539:errorcluster, "data"=w536:T14[], "ref out"=w535:T25)  [unwired: 2 in, 1 out]
                  n90 = case shown="Error .." w539 {
                    selector: w539 -> [w622 _]
                    tunnel: w535 -> [w623 w628]
                    tunnel: [w623 w632] -> w537
                    tunnel: [w622 w630] -> w534
                    tunnel: [w621 w626] -> w532
                    tunnel: w538 -> [_ w631]
                    tunnel: w533 -> [_ w629]
                    tunnel: w536 -> [w621 _]
                    frame No Error {
                      # "New version"
                    }
                    frame Error {
                      # "version 1"
                      n91 = xnode "H5Dread.xnode"("dataset name (this)"=w631, "error in (no error)"=w629, "default"=u16[] [], "ref in"=w628) -> ("error out"=w630:errorcluster, "data"=w625:u16[], "ref out"=w632:i64)  [unwired: 2 in, 1 out]
                      n92 = Array Size(array=w625) -> (size(s)=w624:i32)
                      n93 = call "Get Valid Decay Fit Parameters List.vi"("Parameter ID Array Size"=w624) -> ("Parameter Name Array"=w626:T14[])
                    }
                  }
                  n94 = case shown="Error .." w534 {
                    selector: w534 -> [w694 _]
                    tunnel: w537 -> [w695 w704]
                    tunnel: [w695 w703] -> w563
                    tunnel: [w694 w701] -> w562
                    tunnel: w532 -> [w693 _]
                    tunnel: [w693 w699] -> w561
                    tunnel: "Decay Fit Parameter Names" ("name") -> [_ w702]
                    tunnel: w533 -> [_ w700]
                    frame No Error {
                      # "New version"
                    }
                    frame Error {
                      # "Old version"
                      n95 = xnode "H5Dread.xnode"("dataset name (this)"=w702, "error in (no error)"=w700, "default"=u16[] [], "ref in"=w704) -> ("error out"=w701:errorcluster, "data"=w697:u16[], "ref out"=w703:i64)  [unwired: 2 in, 1 out]
                      n96 = Array Size(array=w697) -> (size(s)=w696:i32)
                      n97 = call "Get Valid Decay Fit Parameters List.vi"("Parameter ID Array Size"=w696) -> ("Parameter Name Array"=w699:T14[])
                    }
                  }
                  n98 = for {
                    tunnel: w561 -> [w781] mode=indexing
                    tunnel: w601 -> [w782]
                    tunnel: [w780] -> w600 mode=indexing
                    n99 = Index Array(array=w782, index=w781) -> (element=w780:string)
                  }
                  n100 = xnode "H5Dread.xnode"("dataset name (this)"="Multiple Decay Fit Parameters Array" ("name"), "error in (no error)"=w562, "default"=w565, "ref in"=w563) -> ("error out"=w556:errorcluster, "data"=w566:dbl[][], "ref out"=w557:T25)  [unwired: 2 in, 1 out]
                  n101 = xnode "H5Dread.xnode"("dataset name (this)"="Decay Preprocessing Parameters" ("name"), "error in (no error)"=w556, "default"=w546, "ref in"=w557) -> ("error out"=w552:errorcluster, "data"=w545:T15, "ref out"=w555:i64)  [unwired: 2 in, 1 out]
                  n102 = xnode "H5Dread.xnode"("dataset name (this)"="Reference Decay: t Array" ("name"), "error in (no error)"=w552, "default"=w543, "ref in"=w555) -> ("error out"=w551:errorcluster, "data"=w542:dbl[], "ref out"=w554:T25)  [unwired: 2 in, 1 out]
                  n103 = xnode "H5Dread.xnode"("dataset name (this)"="Reference Decay: I Array" ("name"), "error in (no error)"=w551, "default"=w541, "ref in"=w554) -> ("error out"=w550:errorcluster, "data"=w540:dbl[], "ref out"=w553:T25)  [unwired: 2 in, 1 out]
                  n104 = Bundle By Name(cluster=w558, "[Multiple Decays Fit Parameters]"=w566, "[Decay Fit Parameter Names]"=w561, "[IRFs]"=w613, "IRF Array Time Axis"=w596, "Fit Options: Decay Preprocessing Parameters"=w545, "Fit Options: Reference Decay.t Array"=w542, "Fit Options: Reference Decay.I Array"=w540) -> (w610:T13)
                  n105 = Array Size(array=w566) -> (size(s)=w595:i32[])
                  n106 = call "Concatenate String Array.vi"("Separator (TAB)"=", ", "String Array"=w600) -> ("Formatted String"=w598:string)  [unwired: 9 in]
                  n107 = xnode "H5Dread.xnode"("dataset name (this)"="Multiple Decay Fit Parameters SDV Array" ("name"), "error in (no error)"=w550, "default"=w565, "ref in"=w553) -> ("error out"=w569:errorcluster, "data"=w564:dbl[][], "ref out"=w568:T25)  [unwired: 2 in, 1 out]
                  n108 = call "Convert Decay Fit Options v1 to v2.vi"("Decay Fit Options v1"=w573) -> ("Decay Fit Options v2"=w530:T24)
                  n109 = Array Size(array=w596) -> (size(s)=w597:i32)
                  n110 = call "Convert Decay Fit Options v2 to v3.vi"("Decay Fit Options v2"=w530) -> ("Decay Fit Options v3"=w529:T2)
                  n111 = Index Array(array=w595) -> (element #1=w594:i32, element #2=w593:i32)  [unwired: 2 in]
                  n112 = Bundle By Name(cluster=w531, "Fit Parameter Constraints"=w574, "Fit Options"=w529, "SYNC Period"=w572) -> (w571:T1)
                  n113 = Format Into String(format string="Parameter Names: %s\nIRFs Length: %d\n# Data Points: %d x %d", initial string=w603, error in=w569, w598, w597, w594, w593) -> (resulting string=w604:string, error out=w605:errorcluster)
                }
                frame "0.4" {
                  w862 = "Decay Fit Parameter IDs" ("name")
                  # "Was Decay Fit Parameter Names previously"
                  n114 = call "AlliGator Read IRFs & Fit Data HDF5 File Metadata.vi"("error in (no error)"=w930, "ref in"=w931) -> ("error out"=w928:errorcluster, "File Metadata"=w925:string, "ref out"=w929:T25)  [unwired: 7 in]
                  n115 = Unbundle By Name(T23 {"SYNC Period"=0.0, "Fit Options"={"Show Fit Residuals"=FALSE, "Fit Model"=enum."1-Exponential", "Residual Type"=enum."Standard", "Max Decay Percentile"=0.0, "Min Decay Percentile"=0.0, "Show Full Decay"=FALSE, "Weights"=enum."Unweighted", "Fitting Method"=enum."Least Square", "Compute Parameter Uncertainties"=FALSE, "Periodic Boundaries"=FALSE, "Model Calculation"=enum."Simulation", "Period"=0.0, "Termination Criteria"={"Max Iterations"=0, "Max Function Calls"=0, "Max Time"=0.0, "Function Tolerance"=0.0, "Parameter Tolerance"=0.0, "Gradient Tolerance"=0.0, "Min Lambda"=0.0, "Max Lambda"=0.0, "Initial Tick Count"=0}, "Offset Resolution"=0.0, "Use Local IRF"=FALSE, "Fitting Algorithm"=enum."Levenberg-Marquardt"}, "Fit Parameter Constraints"=[], "MLE Baseline Offset"=0.0, "MLE Baseline Offset Type"=enum."Absolute"} ("Decay Fit Options & Parameters")) -> ("Fit Parameter Constraints"=w900:T9[], "Fit Options"=w901:T24, "SYNC Period"=w902:dbl[unit], "MLE Baseline Offset Type"=w852:T11, "MLE Baseline Offset"=w846:dbl)
                  n116 = Unbundle By Name(T22 {"IRF Array Time Axis"=[], "[IRFs]"=[], "[Decay Fit Parameter Names]"=[], "[Multiple Decays Fit Parameters]"=[], "Fit Options: Decay Preprocessing Parameters"={"Background Subtraction"=FALSE, "Straighten Decay"=FALSE, "Reverse Gates"=FALSE, "1-Normalized Decay"=FALSE, "Smoothen Decay"=FALSE, "Smoothing Parameter"=0.0, "Shift Decay"=FALSE, "Decay Shift Parameters"={"Type"=enum."Default", "Shift"=0.0, "Threshold"=0.0, "Rotate"=FALSE}, "Extrapolate Decay"=FALSE, "Additional Points"=0, "Head Fraction"=0.0, "Pixel-Normalize Decay"=FALSE, "Use Periodicity"=FALSE, "Use Cursors"=FALSE, "Tail Fraction"=0.0, "Use Decay Pre-Processing"=FALSE, "Fold Decay"=FALSE, "# Folds"=0, "[0-1]-Normalized Decay"=FALSE}, "Fit Options: Reference Decay"={"t Array"=[], "I Array"=[]}} ("IRFs & Fit Data Map")) -> ("[Multiple Decays Fit Parameters]"=w889:dbl[][], "[Decay Fit Parameter Names]"=w883:T14[], "[IRFs]"=w937:dbl[][], "IRF Array Time Axis"=w939:dbl[], "Fit Options: Decay Preprocessing Parameters"=w870:T15, "Fit Options: Reference Decay"=w868:cluster{"t Array":dbl[], "I Array":dbl[]})
                  n117 = call <vilib>:"H5Gclose.vi"("error in (no error)"=w928, "group in"=w929) -> ("error out"=w905:errorcluster)  [unwired: 9 in]
                  n118 = call <vilib>:"H5Gopen.vi"("error in (no error)"=w905, "name"="Decay Fit Options & Parameters" ("dataset name"), "ref in"=w894) -> ("error out"=w914:errorcluster, "group out"=w913:T25)  [unwired: 7 in]
                  n119 = xnode "H5Dread.xnode"("dataset name (this)"="Laser Period" ("dataset name"), "error in (no error)"=w914, "default"=w902, "ref in"=w913) -> ("error out"=w854:errorcluster, "data"=w896:dbl[unit], "ref out"=w851:T25)  [unwired: 2 in, 1 out]
                  n120 = xnode "H5Dread.xnode"("dataset name (this)"="MLE Baseline Offset Type" ("dataset name"), "error in (no error)"=w854, "default"=w852, "ref in"=w851) -> ("error out"=w850:errorcluster, "data"=w845:T11)  [unwired: 2 in, 2 out]
                  n121 = xnode "H5Dread.xnode"("dataset name (this)"="MLE Baseline Offset" ("dataset name"), "error in (no error)"=w850, "default"=w846, "ref in"=w851) -> ("error out"=w848:errorcluster, "data"=w844:dbl, "ref out"=w849:i64)  [unwired: 2 in, 1 out]
                  n122 = xnode "H5Dread.xnode"("dataset name (this)"="Fit Options" ("dataset name"), "error in (no error)"=w848, "default"=w901, "ref in"=w849) -> ("error out"=w912:errorcluster, "data"=w897:T24, "ref out"=w910:i64)  [unwired: 2 in, 1 out]
                  n123 = xnode "H5Dread.xnode"("dataset name (this)"="Fit Parameter Constraints" ("dataset name"), "error in (no error)"=w912, "default"=w900, "ref in"=w910) -> ("error out"=w911:errorcluster, "data"=w898:T9[], "ref out"=w909:T25)  [unwired: 2 in, 1 out]
                  n124 = Unbundle By Name(w868) -> ("t Array"=w867:dbl[], "I Array"=w865:dbl[])
                  n125 = call <vilib>:"H5Gclose.vi"("error in (no error)"=w911, "group in"=w909) -> ("error out"=w904:errorcluster)  [unwired: 9 in]
                  n126 = xnode "H5Dread.xnode"("dataset name (this)"="IRF Array Time Axis" ("dataset name"), "error in (no error)"=w904, "default"=w939, "ref in"=w894) -> ("error out"=w942:errorcluster, "data"=w918:dbl[], "ref out"=w941:T25)  [unwired: 2 in, 1 out]
                  n127 = xnode "H5Dread.xnode"("dataset name (this)"="IRF Array" ("dataset name"), "error in (no error)"=w942, "default"=w937, "ref in"=w941) -> ("error out"=w857:errorcluster, "data"=w935:dbl[][], "ref out"=w934:T25)  [unwired: 2 in, 1 out]
                  n128 = xnode "H5Dread.xnode"("dataset name (this)"=w862, "error in (no error)"=w857, "default"=w883, "ref in"=w934) -> ("error out"=w863:errorcluster, "data"=w860:T14[], "ref out"=w859:T25)  [unwired: 2 in, 1 out]
                  n129 = case shown="Error .." w863 {
                    selector: w863 -> [w974 _]
                    tunnel: w859 -> [w975 w980]
                    tunnel: [w975 w984] -> w861
                    tunnel: [w974 w982] -> w858
                    tunnel: [w973 w978] -> w856
                    tunnel: w862 -> [_ w983]
                    tunnel: w857 -> [_ w981]
                    tunnel: w860 -> [w973 _]
                    frame No Error {
                      # "New version"
                    }
                    frame Error {
                      # "version 1"
                      n130 = xnode "H5Dread.xnode"("dataset name (this)"=w983, "error in (no error)"=w981, "default"=u16[] [], "ref in"=w980) -> ("error out"=w982:errorcluster, "data"=w977:u16[], "ref out"=w984:i64)  [unwired: 2 in, 1 out]
                      n131 = Array Size(array=w977) -> (size(s)=w976:i32)
                      n132 = call "Get Valid Decay Fit Parameters List.vi"("Parameter ID Array Size"=w976) -> ("Parameter Name Array"=w978:T14[])
                    }
                  }
                  n133 = case shown="Error .." w858 {
                    selector: w858 -> [w1046 _]
                    tunnel: w861 -> [w1047 w1056]
                    tunnel: [w1047 w1055] -> w887
                    tunnel: [w1046 w1053] -> w886
                    tunnel: w856 -> [w1045 _]
                    tunnel: [w1045 w1051] -> w885
                    tunnel: "Decay Fit Parameter Names" ("name") -> [_ w1054]
                    tunnel: w857 -> [_ w1052]
                    frame No Error {
                      # "New version"
                    }
                    frame Error {
                      # "Old version"
                      n134 = xnode "H5Dread.xnode"("dataset name (this)"=w1054, "error in (no error)"=w1052, "default"=u16[] [], "ref in"=w1056) -> ("error out"=w1053:errorcluster, "data"=w1049:u16[], "ref out"=w1055:i64)  [unwired: 2 in, 1 out]
                      n135 = Array Size(array=w1049) -> (size(s)=w1048:i32)
                      n136 = call "Get Valid Decay Fit Parameters List.vi"("Parameter ID Array Size"=w1048) -> ("Parameter Name Array"=w1051:T14[])
                    }
                  }
                  n137 = for {
                    tunnel: w885 -> [w1133] mode=indexing
                    tunnel: w923 -> [w1134]
                    tunnel: [w1132] -> w922 mode=indexing
                    n138 = Index Array(array=w1134, index=w1133) -> (element=w1132:string)
                  }
                  n139 = xnode "H5Dread.xnode"("dataset name (this)"="Multiple Decay Fit Parameters Array" ("name"), "error in (no error)"=w886, "default"=w889, "ref in"=w887) -> ("error out"=w880:errorcluster, "data"=w890:dbl[][], "ref out"=w881:T25)  [unwired: 2 in, 1 out]
                  n140 = xnode "H5Dread.xnode"("dataset name (this)"="Decay Preprocessing Parameters" ("name"), "error in (no error)"=w880, "default"=w870, "ref in"=w881) -> ("error out"=w876:errorcluster, "data"=w869:T15, "ref out"=w879:T25)  [unwired: 2 in, 1 out]
                  n141 = xnode "H5Dread.xnode"("dataset name (this)"="Reference Decay: t Array" ("name"), "error in (no error)"=w876, "default"=w867, "ref in"=w879) -> ("error out"=w875:errorcluster, "data"=w866:dbl[], "ref out"=w878:T25)  [unwired: 2 in, 1 out]
                  n142 = xnode "H5Dread.xnode"("dataset name (this)"="Reference Decay: I Array" ("name"), "error in (no error)"=w875, "default"=w865, "ref in"=w878) -> ("error out"=w874:errorcluster, "data"=w864:dbl[], "ref out"=w877:T25)  [unwired: 2 in, 1 out]
                  n143 = Bundle By Name(cluster=w882, "[Multiple Decays Fit Parameters]"=w890, "[Decay Fit Parameter Names]"=w885, "[IRFs]"=w935, "IRF Array Time Axis"=w918, "Fit Options: Decay Preprocessing Parameters"=w869, "Fit Options: Reference Decay.t Array"=w866, "Fit Options: Reference Decay.I Array"=w864) -> (w932:T13)
                  n144 = Array Size(array=w890) -> (size(s)=w917:i32[])
                  n145 = call "Convert Decay Fit Options v2 to v3.vi"("Decay Fit Options v2"=w897) -> ("Decay Fit Options v3"=w843:T2)
                  n146 = call "Concatenate String Array.vi"("Separator (TAB)"=", ", "String Array"=w922) -> ("Formatted String"=w920:string)  [unwired: 9 in]
                  n147 = xnode "H5Dread.xnode"("dataset name (this)"="Multiple Decay Fit Parameters SDV Array" ("name"), "error in (no error)"=w874, "default"=w889, "ref in"=w877) -> ("error out"=w893:errorcluster, "data"=w888:dbl[][], "ref out"=w892:T25)  [unwired: 2 in, 1 out]
                  n148 = Array Size(array=w918) -> (size(s)=w919:i32)
                  n149 = Index Array(array=w917) -> (element #1=w916:i32, element #2=w915:i32)  [unwired: 2 in]
                  n150 = Bundle By Name(cluster=w855, "Fit Parameter Constraints"=w898, "Fit Options"=w843, "SYNC Period"=w896, "MLE Baseline Offset Type"=w845, "MLE Baseline Offset"=w844) -> (w895:T1)
                  n151 = Format Into String(format string="Parameter Names: %s\nIRFs Length: %d\n# Data Points: %d x %d", initial string=w925, error in=w893, w920, w919, w916, w915) -> (resulting string=w926:string, error out=w927:errorcluster)
                }
                frame "0.5" {
                  w1213 = "Decay Fit Parameter IDs" ("name")
                  # "Was Decay Fit Parameter Names previously"
                  n152 = Unbundle By Name(T1 {"SYNC Period"=0.0, "Fit Options"={"Show Fit Residuals"=FALSE, "Fit Model"=enum."1-Exponential", "Residual Type"=enum."Standard", "Max Decay Percentile"=0.0, "Min Decay Percentile"=0.0, "Show Full Decay"=FALSE, "Weights"=enum."Unweighted", "Fitting Method"=enum."Least Square", "Compute Parameter Uncertainties"=FALSE, "Periodic Boundaries"=FALSE, "Model Calculation"=enum."Simulation", "Period"=0.0, "Termination Criteria"={"Max Iterations"=0, "Max Function Calls"=0, "Max Time"=0.0, "Function Tolerance"=0.0, "Parameter Tolerance"=0.0, "Gradient Tolerance"=0.0, "Min Lambda"=0.0, "Max Lambda"=0.0, "Initial Tick Count"=0}, "Offset Resolution"=0.0, "Use Local IRF"=FALSE, "Fitting Algorithm"=enum."Levenberg-Marquardt", "Show Confidence Interval "=TRUE, "Confidence Level"=95.0}, "Fit Parameter Constraints"=[], "MLE Baseline Offset"=0.0, "MLE Baseline Offset Type"=enum."Absolute"} ("Decay Fit Options & Parameters")) -> ("Fit Parameter Constraints"=w1251:T9[], "Fit Options"=w1252:T2, "SYNC Period"=w1253:dbl[unit], "MLE Baseline Offset Type"=w1203:T11, "MLE Baseline Offset"=w1197:dbl)
                  n153 = call "AlliGator Read IRFs & Fit Data HDF5 File Metadata.vi"("error in (no error)"=w1281, "ref in"=w1282) -> ("error out"=w1279:errorcluster, "File Metadata"=w1276:string, "ref out"=w1280:T25)  [unwired: 7 in]
                  n154 = Unbundle By Name(T22 {"IRF Array Time Axis"=[], "[IRFs]"=[], "[Decay Fit Parameter Names]"=[], "[Multiple Decays Fit Parameters]"=[], "Fit Options: Decay Preprocessing Parameters"={"Background Subtraction"=FALSE, "Straighten Decay"=FALSE, "Reverse Gates"=FALSE, "1-Normalized Decay"=FALSE, "Smoothen Decay"=FALSE, "Smoothing Parameter"=0.0, "Shift Decay"=FALSE, "Decay Shift Parameters"={"Type"=enum."Default", "Shift"=0.0, "Threshold"=0.0, "Rotate"=FALSE}, "Extrapolate Decay"=FALSE, "Additional Points"=0, "Head Fraction"=0.0, "Pixel-Normalize Decay"=FALSE, "Use Periodicity"=FALSE, "Use Cursors"=FALSE, "Tail Fraction"=0.0, "Use Decay Pre-Processing"=FALSE, "Fold Decay"=FALSE, "# Folds"=0, "[0-1]-Normalized Decay"=FALSE}, "Fit Options: Reference Decay"={"t Array"=[], "I Array"=[]}} ("IRFs & Fit Data Map")) -> ("[Multiple Decays Fit Parameters]"=w1240:dbl[][], "[Decay Fit Parameter Names]"=w1234:T14[], "[IRFs]"=w1288:dbl[][], "IRF Array Time Axis"=w1290:dbl[], "Fit Options: Decay Preprocessing Parameters"=w1221:T15, "Fit Options: Reference Decay"=w1219:cluster{"t Array":dbl[], "I Array":dbl[]})
                  n155 = call <vilib>:"H5Gclose.vi"("error in (no error)"=w1279, "group in"=w1280) -> ("error out"=w1256:errorcluster)  [unwired: 9 in]
                  n156 = call <vilib>:"H5Gopen.vi"("error in (no error)"=w1256, "name"="Decay Fit Options & Parameters" ("dataset name"), "ref in"=w1245) -> ("error out"=w1265:errorcluster, "group out"=w1264:T25)  [unwired: 7 in]
                  n157 = xnode "H5Dread.xnode"("dataset name (this)"="Laser Period" ("dataset name"), "error in (no error)"=w1265, "default"=w1253, "ref in"=w1264) -> ("error out"=w1205:errorcluster, "data"=w1247:dbl[unit], "ref out"=w1202:T25)  [unwired: 2 in, 1 out]
                  n158 = xnode "H5Dread.xnode"("dataset name (this)"="MLE Baseline Offset Type" ("dataset name"), "error in (no error)"=w1205, "default"=w1203, "ref in"=w1202) -> ("error out"=w1201:errorcluster, "data"=w1196:T11)  [unwired: 2 in, 2 out]
                  n159 = xnode "H5Dread.xnode"("dataset name (this)"="MLE Baseline Offset" ("dataset name"), "error in (no error)"=w1201, "default"=w1197, "ref in"=w1202) -> ("error out"=w1199:errorcluster, "data"=w1195:dbl, "ref out"=w1200:i64)  [unwired: 2 in, 1 out]
                  n160 = xnode "H5Dread.xnode"("dataset name (this)"="Fit Options" ("dataset name"), "error in (no error)"=w1199, "default"=w1252, "ref in"=w1200) -> ("error out"=w1263:errorcluster, "data"=w1248:T2, "ref out"=w1261:i64)  [unwired: 2 in, 1 out]
                  n161 = xnode "H5Dread.xnode"("dataset name (this)"="Fit Parameter Constraints" ("dataset name"), "error in (no error)"=w1263, "default"=w1251, "ref in"=w1261) -> ("error out"=w1262:errorcluster, "data"=w1249:T9[], "ref out"=w1260:T25)  [unwired: 2 in, 1 out]
                  n162 = Unbundle By Name(w1219) -> ("t Array"=w1218:dbl[], "I Array"=w1216:dbl[])
                  n163 = call <vilib>:"H5Gclose.vi"("error in (no error)"=w1262, "group in"=w1260) -> ("error out"=w1255:errorcluster)  [unwired: 9 in]
                  n164 = xnode "H5Dread.xnode"("dataset name (this)"="IRF Array Time Axis" ("dataset name"), "error in (no error)"=w1255, "default"=w1290, "ref in"=w1245) -> ("error out"=w1293:errorcluster, "data"=w1269:dbl[], "ref out"=w1292:T25)  [unwired: 2 in, 1 out]
                  n165 = xnode "H5Dread.xnode"("dataset name (this)"="IRF Array" ("dataset name"), "error in (no error)"=w1293, "default"=w1288, "ref in"=w1292) -> ("error out"=w1208:errorcluster, "data"=w1286:dbl[][], "ref out"=w1285:T25)  [unwired: 2 in, 1 out]
                  n166 = xnode "H5Dread.xnode"("dataset name (this)"=w1213, "error in (no error)"=w1208, "default"=w1234, "ref in"=w1285) -> ("error out"=w1214:errorcluster, "data"=w1211:T14[], "ref out"=w1210:T25)  [unwired: 2 in, 1 out]
                  n167 = case shown="Error .." w1214 {
                    selector: w1214 -> [w1325 _]
                    tunnel: w1210 -> [w1326 w1331]
                    tunnel: [w1326 w1335] -> w1212
                    tunnel: [w1325 w1333] -> w1209
                    tunnel: [w1324 w1329] -> w1207
                    tunnel: w1213 -> [_ w1334]
                    tunnel: w1208 -> [_ w1332]
                    tunnel: w1211 -> [w1324 _]
                    frame No Error {
                      # "New version"
                    }
                    frame Error {
                      # "version 1"
                      n168 = xnode "H5Dread.xnode"("dataset name (this)"=w1334, "error in (no error)"=w1332, "default"=u16[] [], "ref in"=w1331) -> ("error out"=w1333:errorcluster, "data"=w1328:u16[], "ref out"=w1335:i64)  [unwired: 2 in, 1 out]
                      n169 = Array Size(array=w1328) -> (size(s)=w1327:i32)
                      n170 = call "Get Valid Decay Fit Parameters List.vi"("Parameter ID Array Size"=w1327) -> ("Parameter Name Array"=w1329:T14[])
                    }
                  }
                  n171 = case shown="Error .." w1209 {
                    selector: w1209 -> [w1397 _]
                    tunnel: w1212 -> [w1398 w1407]
                    tunnel: [w1398 w1406] -> w1238
                    tunnel: [w1397 w1404] -> w1237
                    tunnel: w1207 -> [w1396 _]
                    tunnel: [w1396 w1402] -> w1236
                    tunnel: "Decay Fit Parameter Names" ("name") -> [_ w1405]
                    tunnel: w1208 -> [_ w1403]
                    frame No Error {
                      # "New version"
                    }
                    frame Error {
                      # "Old version"
                      n172 = xnode "H5Dread.xnode"("dataset name (this)"=w1405, "error in (no error)"=w1403, "default"=u16[] [], "ref in"=w1407) -> ("error out"=w1404:errorcluster, "data"=w1400:u16[], "ref out"=w1406:i64)  [unwired: 2 in, 1 out]
                      n173 = Array Size(array=w1400) -> (size(s)=w1399:i32)
                      n174 = call "Get Valid Decay Fit Parameters List.vi"("Parameter ID Array Size"=w1399) -> ("Parameter Name Array"=w1402:T14[])
                    }
                  }
                  n175 = for {
                    tunnel: w1236 -> [w1484] mode=indexing
                    tunnel: w1274 -> [w1485]
                    tunnel: [w1483] -> w1273 mode=indexing
                    n176 = Index Array(array=w1485, index=w1484) -> (element=w1483:string)
                  }
                  n177 = xnode "H5Dread.xnode"("dataset name (this)"="Multiple Decay Fit Parameters Array" ("name"), "error in (no error)"=w1237, "default"=w1240, "ref in"=w1238) -> ("error out"=w1231:errorcluster, "data"=w1241:dbl[][], "ref out"=w1232:T25)  [unwired: 2 in, 1 out]
                  n178 = xnode "H5Dread.xnode"("dataset name (this)"="Decay Preprocessing Parameters" ("name"), "error in (no error)"=w1231, "default"=w1221, "ref in"=w1232) -> ("error out"=w1227:errorcluster, "data"=w1220:T15, "ref out"=w1230:T25)  [unwired: 2 in, 1 out]
                  n179 = xnode "H5Dread.xnode"("dataset name (this)"="Reference Decay: t Array" ("name"), "error in (no error)"=w1227, "default"=w1218, "ref in"=w1230) -> ("error out"=w1226:errorcluster, "data"=w1217:dbl[], "ref out"=w1229:T25)  [unwired: 2 in, 1 out]
                  n180 = xnode "H5Dread.xnode"("dataset name (this)"="Reference Decay: I Array" ("name"), "error in (no error)"=w1226, "default"=w1216, "ref in"=w1229) -> ("error out"=w1225:errorcluster, "data"=w1215:dbl[], "ref out"=w1228:T25)  [unwired: 2 in, 1 out]
                  n181 = Bundle By Name(cluster=w1233, "[Multiple Decays Fit Parameters]"=w1241, "[Decay Fit Parameter Names]"=w1236, "[IRFs]"=w1286, "IRF Array Time Axis"=w1269, "Fit Options: Decay Preprocessing Parameters"=w1220, "Fit Options: Reference Decay.t Array"=w1217, "Fit Options: Reference Decay.I Array"=w1215) -> (w1283:T13)
                  n182 = Array Size(array=w1241) -> (size(s)=w1268:i32[])
                  n183 = call "Concatenate String Array.vi"("Separator (TAB)"=", ", "String Array"=w1273) -> ("Formatted String"=w1271:string)  [unwired: 9 in]
                  n184 = xnode "H5Dread.xnode"("dataset name (this)"="Multiple Decay Fit Parameters SDV Array" ("name"), "error in (no error)"=w1225, "default"=w1240, "ref in"=w1228) -> ("error out"=w1244:errorcluster, "data"=w1239:dbl[][], "ref out"=w1243:T25)  [unwired: 2 in, 1 out]
                  n185 = Array Size(array=w1269) -> (size(s)=w1270:i32)
                  n186 = Index Array(array=w1268) -> (element #1=w1267:i32, element #2=w1266:i32)  [unwired: 2 in]
                  n187 = Bundle By Name(cluster=w1206, "Fit Parameter Constraints"=w1249, "Fit Options"=w1248, "SYNC Period"=w1247, "MLE Baseline Offset Type"=w1196, "MLE Baseline Offset"=w1195) -> (w1246:T1)
                  n188 = Format Into String(format string="Parameter Names: %s\nIRFs Length: %d\n# Data Points: %d x %d", initial string=w1276, error in=w1244, w1271, w1270, w1267, w1266) -> (resulting string=w1277:string, error out=w1278:errorcluster)
                }
                frame "0.6" {
                  w1571 = "Decay Fit Parameter IDs" ("name")
                  # "Was Decay Fit Parameter Names previously"
                  n189 = Unbundle By Name(T1 {"SYNC Period"=0.0, "Fit Options"={"Show Fit Residuals"=FALSE, "Fit Model"=enum."1-Exponential", "Residual Type"=enum."Standard", "Max Decay Percentile"=0.0, "Min Decay Percentile"=0.0, "Show Full Decay"=FALSE, "Weights"=enum."Unweighted", "Fitting Method"=enum."Least Square", "Compute Parameter Uncertainties"=FALSE, "Periodic Boundaries"=FALSE, "Model Calculation"=enum."Simulation", "Period"=0.0, "Termination Criteria"={"Max Iterations"=0, "Max Function Calls"=0, "Max Time"=0.0, "Function Tolerance"=0.0, "Parameter Tolerance"=0.0, "Gradient Tolerance"=0.0, "Min Lambda"=0.0, "Max Lambda"=0.0, "Initial Tick Count"=0}, "Offset Resolution"=0.0, "Use Local IRF"=FALSE, "Fitting Algorithm"=enum."Levenberg-Marquardt", "Show Confidence Interval "=TRUE, "Confidence Level"=95.0}, "Fit Parameter Constraints"=[], "MLE Baseline Offset"=0.0, "MLE Baseline Offset Type"=enum."Absolute"} ("Decay Fit Options & Parameters")) -> ("Fit Parameter Constraints"=w1607:T9[], "Fit Options"=w1608:T2, "SYNC Period"=w1609:dbl[unit], "MLE Baseline Offset Type"=w1561:T11, "MLE Baseline Offset"=w1555:dbl)
                  n190 = call "AlliGator Read IRFs & Fit Data HDF5 File Metadata.vi"("error in (no error)"=w1637, "ref in"=w1638) -> ("error out"=w1635:errorcluster, "File Metadata"=w1632:string, "ref out"=w1636:T25)  [unwired: 7 in]
                  n191 = Unbundle By Name(T13 {"IRF Array Time Axis"=[], "[IRFs]"=[], "[Decay Fit Parameter Names]"=[], "[Multiple Decays Fit Parameters]"=[], "Fit Options: Decay Preprocessing Parameters"={"Background Subtraction"=FALSE, "Straighten Decay"=FALSE, "Reverse Gates"=FALSE, "1-Normalized Decay"=FALSE, "Smoothen Decay"=FALSE, "Smoothing Parameter"=0.0, "Shift Decay"=FALSE, "Decay Shift Parameters"={"Type"=enum."Default", "Shift"=0.0, "Threshold"=0.0, "Rotate"=FALSE}, "Extrapolate Decay"=FALSE, "Additional Points"=0, "Head Fraction"=0.0, "Pixel-Normalize Decay"=FALSE, "Use Periodicity"=FALSE, "Use Cursors"=FALSE, "Tail Fraction"=0.0, "Use Decay Pre-Processing"=FALSE, "Fold Decay"=FALSE, "# Folds"=0, "[0-1]-Normalized Decay"=FALSE}, "Fit Options: Reference Decay"={"t Array"=[], "I Array"=[]}, "[Decay Sum]"=[]} ("IRFs & Fit Data Map")) -> ("[Multiple Decays Fit Parameters]"=w1596:dbl[][], "[Decay Fit Parameter Names]"=w1590:T14[], "[IRFs]"=w1644:dbl[][], "IRF Array Time Axis"=w1646:dbl[], "Fit Options: Decay Preprocessing Parameters"=w1579:T15, "Fit Options: Reference Decay"=w1577:cluster{"t Array":dbl[], "I Array":dbl[]}, "[Decay Sum]"=w1547:dbl[])
                  n192 = call <vilib>:"H5Gclose.vi"("error in (no error)"=w1635, "group in"=w1636) -> ("error out"=w1612:errorcluster)  [unwired: 9 in]
                  n193 = call <vilib>:"H5Gopen.vi"("error in (no error)"=w1612, "name"="Decay Fit Options & Parameters" ("dataset name"), "ref in"=w1601) -> ("error out"=w1621:errorcluster, "group out"=w1620:T25)  [unwired: 7 in]
                  n194 = xnode "H5Dread.xnode"("dataset name (this)"="Laser Period" ("dataset name"), "error in (no error)"=w1621, "default"=w1609, "ref in"=w1620) -> ("error out"=w1563:errorcluster, "data"=w1603:dbl[unit], "ref out"=w1560:T25)  [unwired: 2 in, 1 out]
                  n195 = xnode "H5Dread.xnode"("dataset name (this)"="MLE Baseline Offset Type" ("dataset name"), "error in (no error)"=w1563, "default"=w1561, "ref in"=w1560) -> ("error out"=w1559:errorcluster, "data"=w1554:T11)  [unwired: 2 in, 2 out]
                  n196 = xnode "H5Dread.xnode"("dataset name (this)"="MLE Baseline Offset" ("dataset name"), "error in (no error)"=w1559, "default"=w1555, "ref in"=w1560) -> ("error out"=w1557:errorcluster, "data"=w1553:dbl, "ref out"=w1558:i64)  [unwired: 2 in, 1 out]
                  n197 = xnode "H5Dread.xnode"("dataset name (this)"="Fit Options" ("dataset name"), "error in (no error)"=w1557, "default"=w1608, "ref in"=w1558) -> ("error out"=w1619:errorcluster, "data"=w1604:T2, "ref out"=w1617:i64)  [unwired: 2 in, 1 out]
                  n198 = xnode "H5Dread.xnode"("dataset name (this)"="Fit Parameter Constraints" ("dataset name"), "error in (no error)"=w1619, "default"=w1607, "ref in"=w1617) -> ("error out"=w1618:errorcluster, "data"=w1605:T9[], "ref out"=w1616:T25)  [unwired: 2 in, 1 out]
                  n199 = Unbundle By Name(w1577) -> ("t Array"=w1576:dbl[], "I Array"=w1574:dbl[])
                  n200 = call <vilib>:"H5Gclose.vi"("error in (no error)"=w1618, "group in"=w1616) -> ("error out"=w1611:errorcluster)  [unwired: 9 in]
                  n201 = xnode "H5Dread.xnode"("dataset name (this)"="IRF Array Time Axis" ("dataset name"), "error in (no error)"=w1611, "default"=w1646, "ref in"=w1601) -> ("error out"=w1649:errorcluster, "data"=w1625:dbl[], "ref out"=w1648:T25)  [unwired: 2 in, 1 out]
                  n202 = xnode "H5Dread.xnode"("dataset name (this)"="IRF Array" ("dataset name"), "error in (no error)"=w1649, "default"=w1644, "ref in"=w1648) -> ("error out"=w1566:errorcluster, "data"=w1642:dbl[][], "ref out"=w1641:T25)  [unwired: 2 in, 1 out]
                  n203 = xnode "H5Dread.xnode"("dataset name (this)"=w1571, "error in (no error)"=w1566, "default"=w1590, "ref in"=w1641) -> ("error out"=w1572:errorcluster, "data"=w1569:T14[], "ref out"=w1568:T25)  [unwired: 2 in, 1 out]
                  n204 = case shown="Error .." w1572 {
                    selector: w1572 -> [w1696 _]
                    tunnel: w1568 -> [w1697 w1702]
                    tunnel: [w1697 w1706] -> w1570
                    tunnel: [w1696 w1704] -> w1567
                    tunnel: [w1695 w1700] -> w1565
                    tunnel: w1571 -> [_ w1705]
                    tunnel: w1566 -> [_ w1703]
                    tunnel: w1569 -> [w1695 _]
                    frame No Error {
                      # "New version"
                    }
                    frame Error {
                      # "version 1"
                      n205 = xnode "H5Dread.xnode"("dataset name (this)"=w1705, "error in (no error)"=w1703, "default"=u16[] [], "ref in"=w1702) -> ("error out"=w1704:errorcluster, "data"=w1699:u16[], "ref out"=w1706:i64)  [unwired: 2 in, 1 out]
                      n206 = Array Size(array=w1699) -> (size(s)=w1698:i32)
                      n207 = call "Get Valid Decay Fit Parameters List.vi"("Parameter ID Array Size"=w1698) -> ("Parameter Name Array"=w1700:T14[])
                    }
                  }
                  n208 = case shown="Error .." w1567 {
                    selector: w1567 -> [w1768 _]
                    tunnel: w1570 -> [w1769 w1778]
                    tunnel: [w1769 w1777] -> w1594
                    tunnel: [w1768 w1775] -> w1593
                    tunnel: w1565 -> [w1767 _]
                    tunnel: [w1767 w1773] -> w1592
                    tunnel: "Decay Fit Parameter Names" ("name") -> [_ w1776]
                    tunnel: w1566 -> [_ w1774]
                    frame No Error {
                      # "New version"
                    }
                    frame Error {
                      # "Old version"
                      n209 = xnode "H5Dread.xnode"("dataset name (this)"=w1776, "error in (no error)"=w1774, "default"=u16[] [], "ref in"=w1778) -> ("error out"=w1775:errorcluster, "data"=w1771:u16[], "ref out"=w1777:i64)  [unwired: 2 in, 1 out]
                      n210 = Array Size(array=w1771) -> (size(s)=w1770:i32)
                      n211 = call "Get Valid Decay Fit Parameters List.vi"("Parameter ID Array Size"=w1770) -> ("Parameter Name Array"=w1773:T14[])
                    }
                  }
                  n212 = for {
                    tunnel: w1592 -> [w1855] mode=indexing
                    tunnel: w1630 -> [w1856]
                    tunnel: [w1854] -> w1629 mode=indexing
                    n213 = Index Array(array=w1856, index=w1855) -> (element=w1854:string)
                  }
                  n214 = xnode "H5Dread.xnode"("dataset name (this)"="Multiple Decay Fit Parameters Array" ("name"), "error in (no error)"=w1593, "default"=w1596, "ref in"=w1594) -> ("error out"=w1587:errorcluster, "data"=w1597:dbl[][], "ref out"=w1588:T25)  [unwired: 2 in, 1 out]
                  n215 = xnode "H5Dread.xnode"("dataset name (this)"="Decay Preprocessing Parameters" ("name"), "error in (no error)"=w1587, "default"=w1579, "ref in"=w1588) -> ("error out"=w1584:errorcluster, "data"=w1578:T15, "ref out"=w1586:T25)  [unwired: 2 in, 1 out]
                  n216 = xnode "H5Dread.xnode"("dataset name (this)"="Reference Decay: t Array" ("name"), "error in (no error)"=w1584, "default"=w1576, "ref in"=w1586) -> ("error out"=w1583:errorcluster, "data"=w1575:dbl[], "ref out"=w1585:T25)  [unwired: 2 in, 1 out]
                  n217 = xnode "H5Dread.xnode"("dataset name (this)"="Reference Decay: I Array" ("name"), "error in (no error)"=w1583, "default"=w1574, "ref in"=w1585) -> ("error out"=w1551:errorcluster, "data"=w1573:dbl[], "ref out"=w1552:T25)  [unwired: 2 in, 1 out]
                  n218 = xnode "H5Dread.xnode"("dataset name (this)"="Decay Sums" ("name"), "error in (no error)"=w1551, "default"=w1547, "ref in"=w1552) -> ("error out"=w1549:errorcluster, "data"=w1546:dbl[], "ref out"=w1550:i64)  [unwired: 2 in, 1 out]
                  n219 = Bundle By Name(cluster=w1589, "[Multiple Decays Fit Parameters]"=w1597, "[Decay Fit Parameter Names]"=w1592, "[IRFs]"=w1642, "IRF Array Time Axis"=w1625, "Fit Options: Decay Preprocessing Parameters"=w1578, "Fit Options: Reference Decay.t Array"=w1575, "Fit Options: Reference Decay.I Array"=w1573, "[Decay Sum]"=w1546) -> (w1639:T13)
                  n220 = Array Size(array=w1597) -> (size(s)=w1624:i32[])
                  n221 = call "Concatenate String Array.vi"("Separator (TAB)"=", ", "String Array"=w1629) -> ("Formatted String"=w1627:string)  [unwired: 9 in]
                  n222 = xnode "H5Dread.xnode"("dataset name (this)"="Multiple Decay Fit Parameters SDV Array" ("name"), "error in (no error)"=w1549, "default"=w1596, "ref in"=w1550) -> ("error out"=w1600:errorcluster, "data"=w1595:dbl[][], "ref out"=w1599:T25)  [unwired: 2 in, 1 out]
                  n223 = Array Size(array=w1625) -> (size(s)=w1626:i32)
                  n224 = Index Array(array=w1624) -> (element #1=w1623:i32, element #2=w1622:i32)  [unwired: 2 in]
                  n225 = Bundle By Name(cluster=w1564, "Fit Parameter Constraints"=w1605, "Fit Options"=w1604, "SYNC Period"=w1603, "MLE Baseline Offset Type"=w1554, "MLE Baseline Offset"=w1553) -> (w1602:T1)
                  n226 = Format Into String(format string="Parameter Names: %s\nIRFs Length: %d\n# Data Points: %d x %d", initial string=w1632, error in=w1600, w1627, w1626, w1623, w1622) -> (resulting string=w1633:string, error out=w1634:errorcluster)
                }
              }
            }
            frame True {
              # "File Type & Version only"
              n227 = call <vilib>:"H5Gclose.vi"("error in (no error)"=w1920, "group in"=w1919) -> ("error out"=w1917:errorcluster)  [unwired: 9 in]
            }
          }
        }
      }
      n228 = call <vilib>:"H5Fclose.vi"("error in (no error)"=w41, "ref"=w42) -> ("error out"=w25:errorcluster)  [unwired: 9 in]
      n229 = call "High Resolution Timing.vi"("relative seconds (NaN)"=w38, "Error In"=w25) -> ("elapsed (relative) seconds"=w37:dbl, "Error Out"=w39:errorcluster)  [unwired: 15 in, 1 out]
    }
  }
  "error out" <- w13
  "elapsed (relative) seconds" <- w6
  "Data Description" <- w4
  "IRFs & Fit Data Map v3" <- w5
  "Decay Fit Options & Parameters" <- w3
  "[Multiple Decays Fit Parameters SDV]" <- w1
